vi "Test_waveform.vi"() -> ()   [LabVIEW 2017]
uses:
  Range_Shunt_selector.ctl
  <vilib>/Waveform/WDTFileIO.llb/ Write Waveform to File.vi
  <vilib>/Waveform/WDTFileIO.llb/Read Waveform from File.vi
  <vilib>/Utility/config.llb/Write Key (I32).vi
  <vilib>/Utility/config.llb/Write Key (Boolean).vi
  <vilib>/Utility/config.llb/Read Key (I32).vi
  <vilib>/Utility/config.llb/Read Key (Boolean).vi
  <vilib>/measure/madcrms.llb/Basic Averaged DC-RMS for 1 Chan.vi
  <resource>/objmgr/daqmx.rc
  <vilib>/Utility/config.llb/NI_LVConfig.lvlib
  <vilib>/measure/NI_MAPro.lvlib
panel:
  out "current time":timestamp
  out "Samples":i32=20000
  out "error out 3":errorcluster
  out "PhysicalChanName":tag
  out "DEV SN":u32 format="%.0x"
  out "mARange":dbl
  out "Boolean":bool
  out "DevSerialNum":u32
  in  "uA_bank0":dbl=1.5 format="%#_13g"
  out "Task out":refnum<k21>="Stop"
  out "Sample rate":dbl=20000.0 format="%#_13g"
  out "Clear":bool=TRUE
  out "Ver":string
  out "seconds since 1Jan1904":timestamp
  in  "Tab Control":enum32{"Current Tracking", "Logging"}(tab)
  out "Save":bool
  out "Total Time":string
  in  "Sampling Rate":T1(ring)
  out "out_range":bool
  in  "Save setting":bool
  out "PW_Source":bool
  out "EX_IN_INdicator":bool
  out "Lable.Unit_VOl_MA_UA":string
  in  "Ext PW Vol Monitor":bool
  out "POWER ON_OFF":bool
  out "vbat_lb":dbl format="%#_4f"
  in  "bypass Shunt":bool
  in  "Internal PW":bool
  in  "USB":tag="Dev1"
  out "schematic":bool
  in  "Save":bool
  in  "Load":bool
  in  "Calib":bool
  in  "Power ON/OFF":bool
  in  "Profile":enum16{"SAM", "DIANA", "Hi-POWER", "Other..."}(ring)
  in  "Take Picture":bool
  in  "Orginal":bool
  in  "Clear Graph":bool
  in  "ZOOM M1M2":bool
  in  "ZOOM -":bool
  in  "ZOOM +":bool
  in  "stop":bool
  out "Vbat":dbl format="%#.3f"
  in  "Measure":bool
  in  "Range - Shunts":T2
  out "PW_Internal_Source":dbl
  out "Min":dbl
  out "Max":dbl
  out "Delta(s)":sgl
  in  "Center":bool
  out "Avg":dbl
  out "Waveform_main":waveform(sgl)(graph)
  out "Waveform_sub":waveform(dbl)(graph)
  out "Average (uA)":dbl caption="Average (mA)" format="%#_6f"
  in  "Vout  - Vbat profile":enum16{"3.8VDC", "2.9VDC", "By Pass", "4.0VDC"}(ring)=enum."2.9VDC" caption="Vout  - Vbat"
  # "µPower kit for Wear OS Dev"
  # "Vbat"
  # "Vdut- Vbat"
  # "DUT"
  # "Rs"
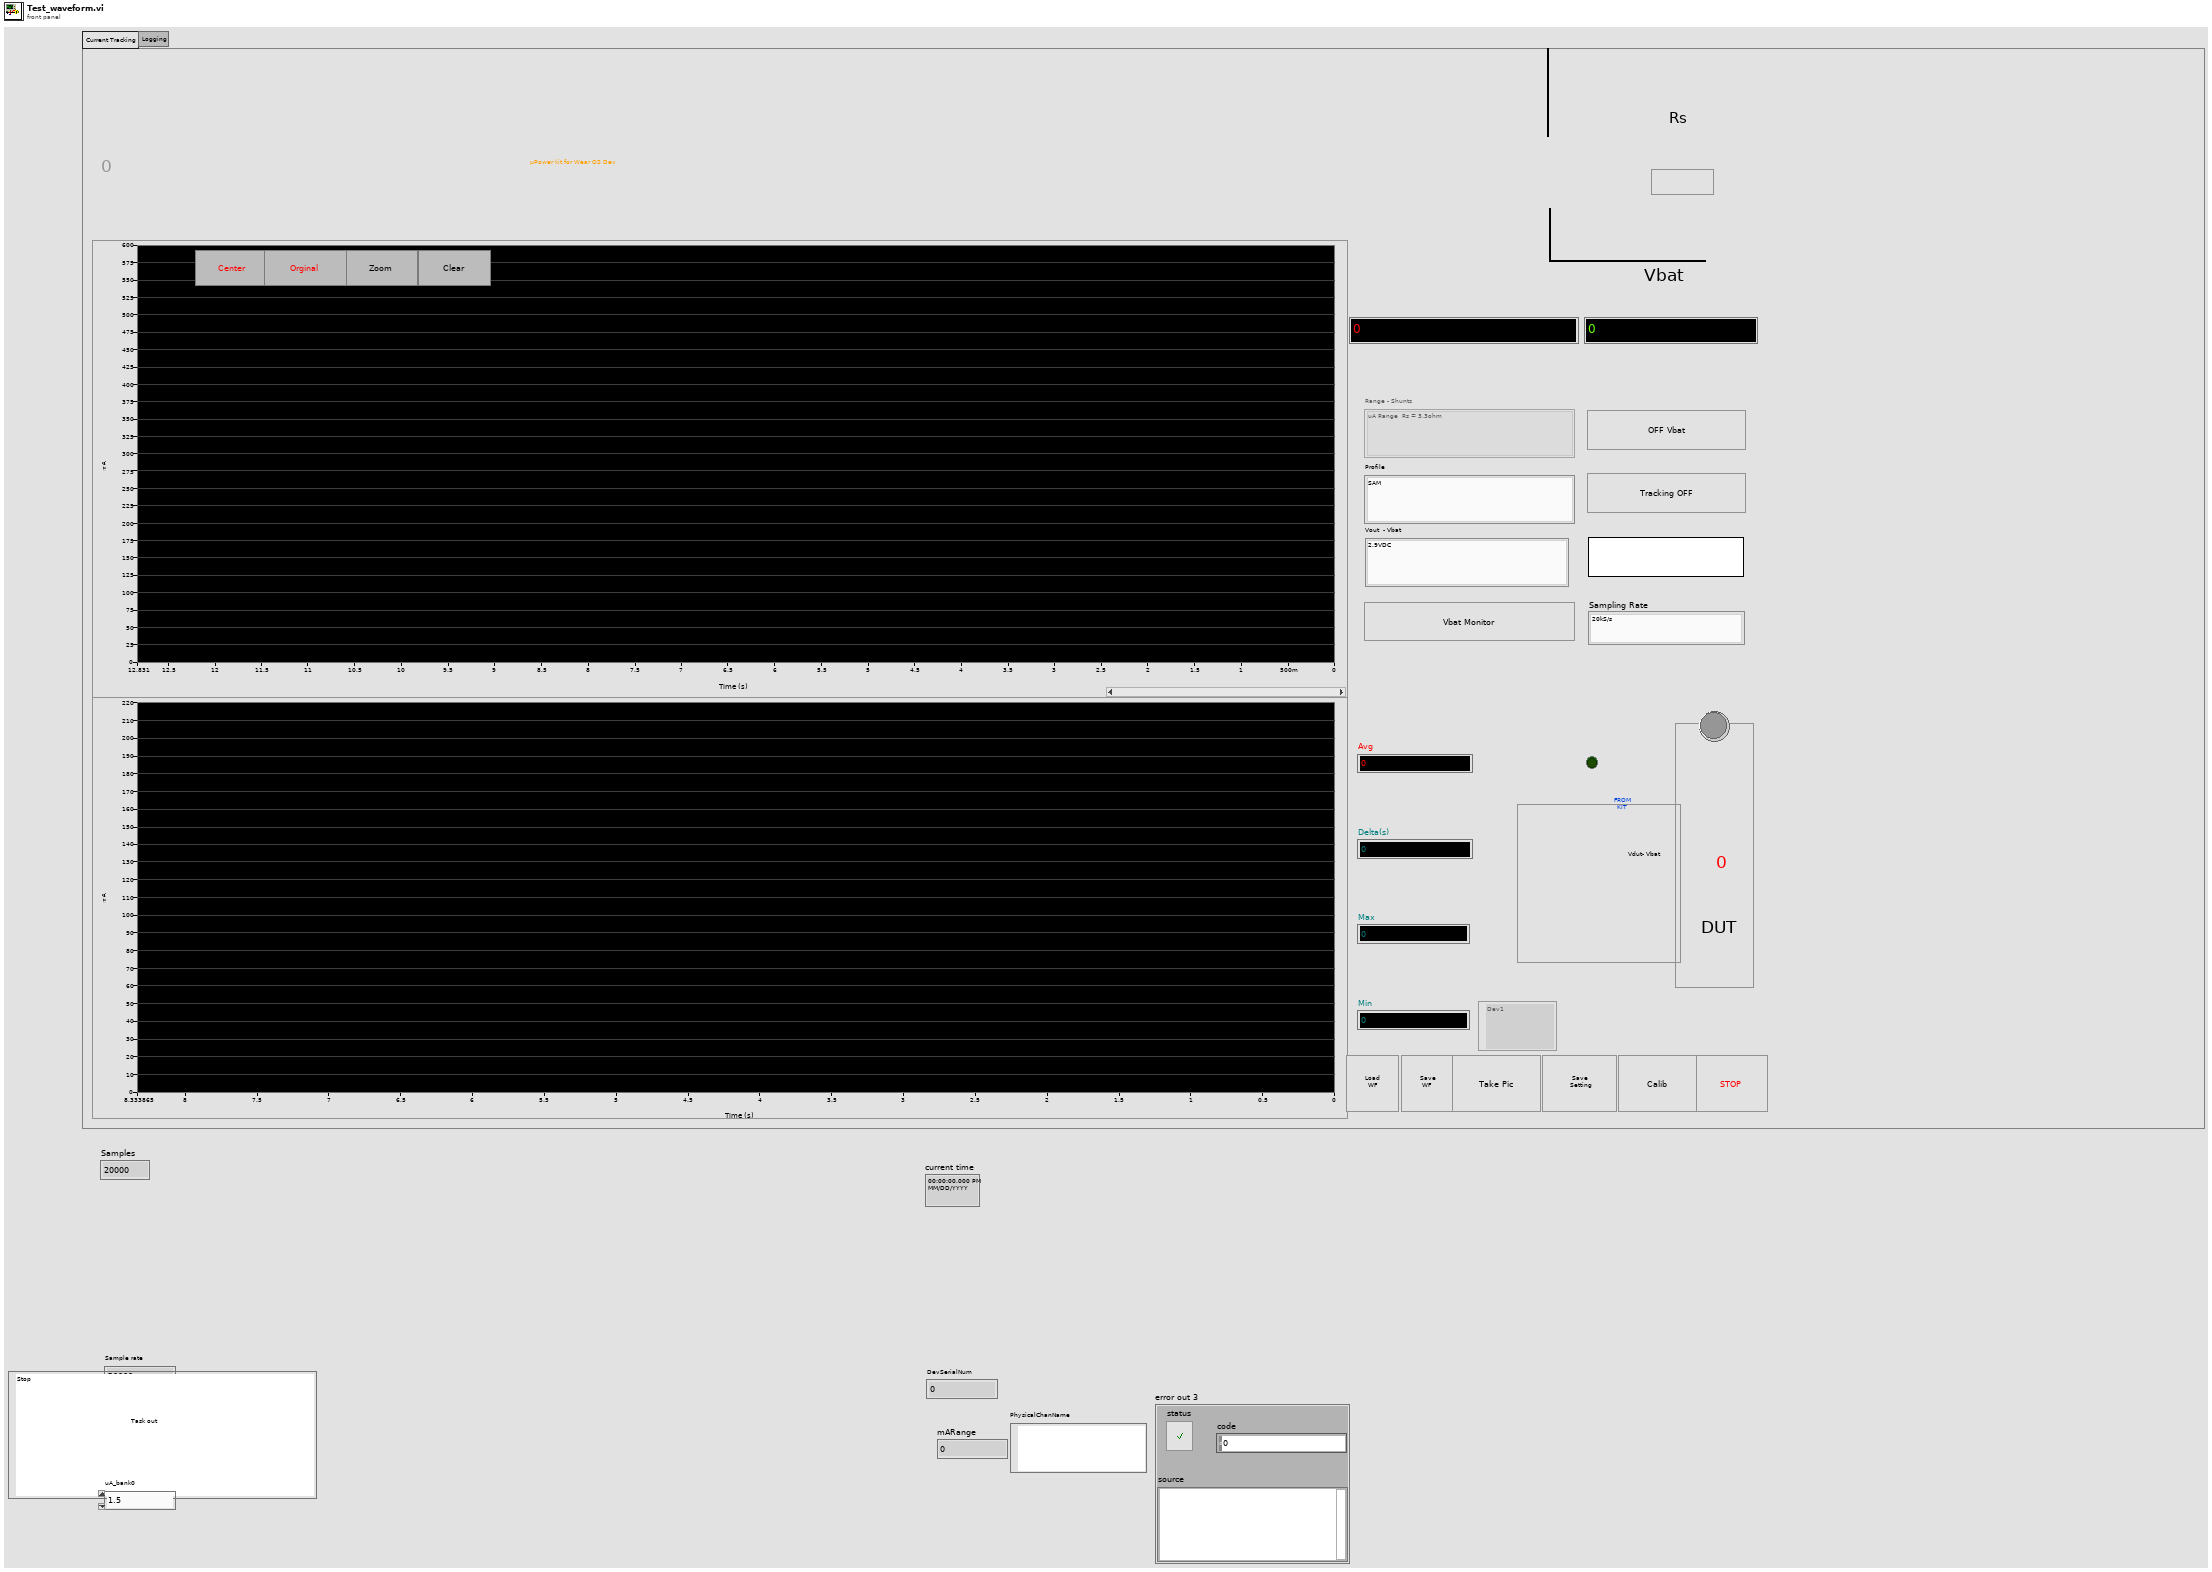
[diagram p1: front panel]
types:
  T1 = enum16{"20kS/s", "10kS/s", "5kS/s", "2kS/s", "1kS/s", "500S/s", "100S/s"}
  T2 = typedef "Range_Shunt_selector.ctl" = enum16{"uA Range  Rs = 3.3ohm", "mA Range Rs = 3.3ohm", "mA Range Rs = 1ohm", "mA Range Rs = 1ohm - X2"}
  T3 = enum8{"Enabled", "Disabled", "Disabled and Grayed Out"}
  T4 = typedef "NI_LVConfig.lvlib/Config Data RefNum.ctl" = refnum<k1>
  T5 = enum16{"Internal PW Source", "External PW Source"}
  T6 = enum16{"Turn On bypass - Off Shunt", "Turn Off bypass - On Shunt"}
  T7 = typedef "LVCursorListTypeDef.ctl" = cluster{"Name":string, "Color":u32, "Style":u8, "Point Style":u8, "Name Visible":bool, "Allow Drag":bool, "Cursor Mode":u32, "Plot":i32, "Index":i32, "Position":cluster{"X":dbl, "Y":dbl}, "X Scale":u32, "Y Scale":u32, "Watch Plots":i32[], "Watch All Plots":bool, "Plot Area":i32, "Label Offset":cluster{"X":dbl, "Y":dbl}}[]
  T8 = typedef "imagedata.ctl" = cluster{"image type":i32, "image depth":i32, "image":u8[], "mask":u8[], "colors":u32[], "Rectangle":cluster{"left":i16, "top":i16, "right":i16, "bottom":i16}}
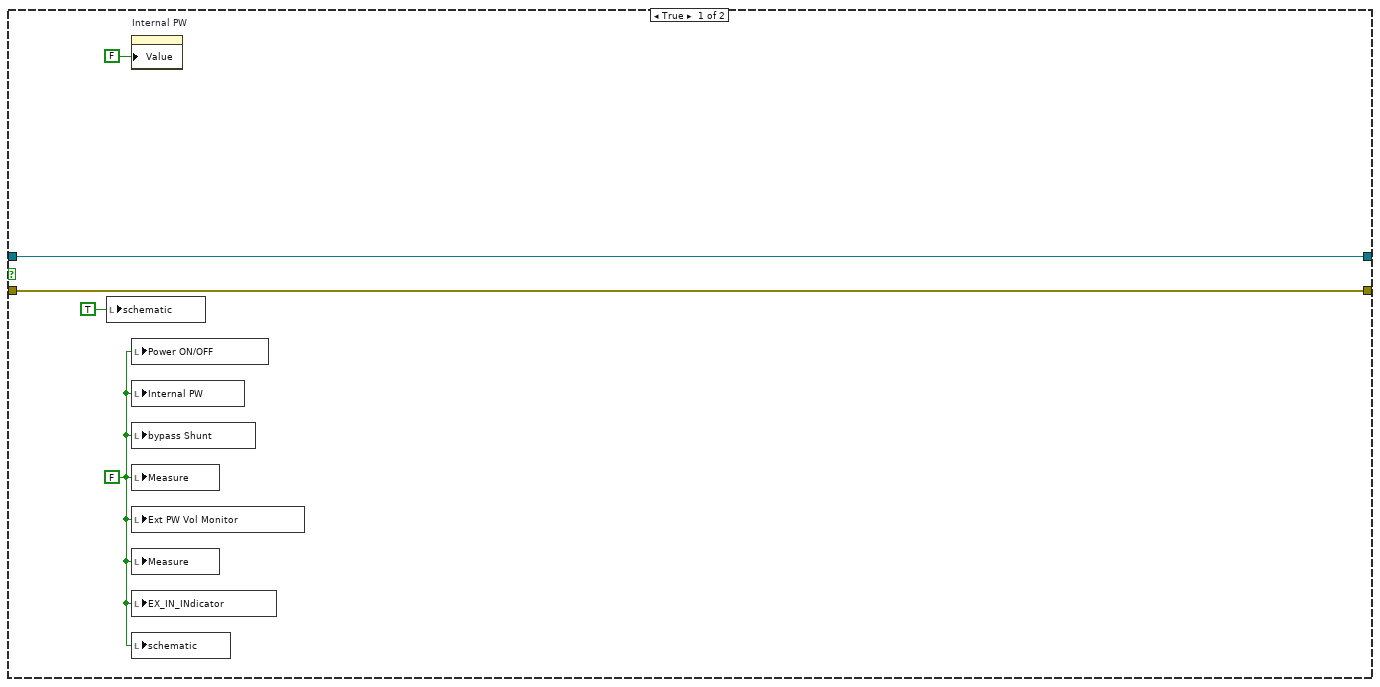
[diagram p2: hidden frame]
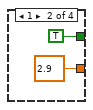
[diagram p3: hidden frame]
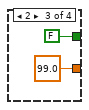
[diagram p4: hidden frame]
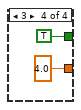
[diagram p5: hidden frame]
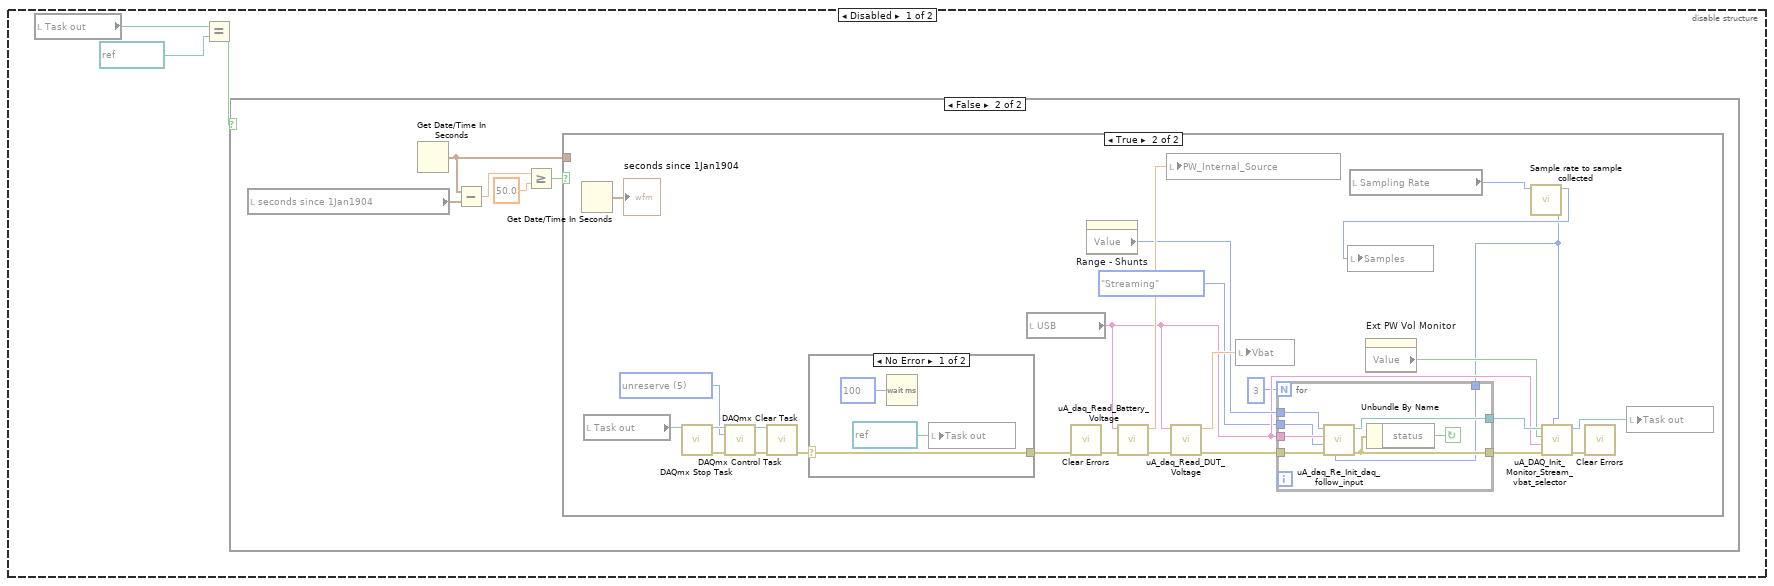
[diagram p7: hidden frame]
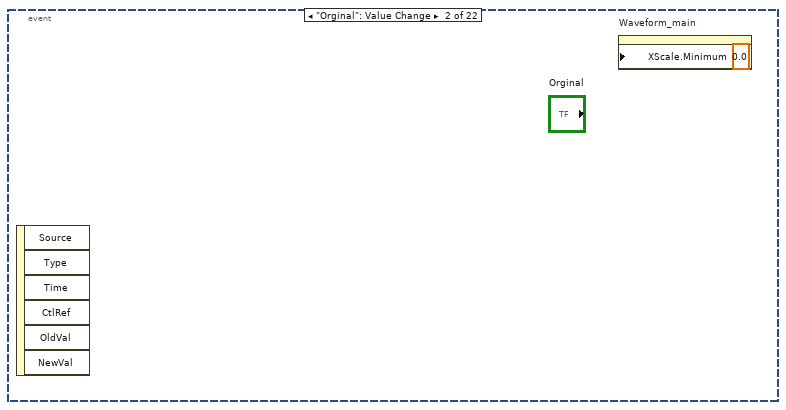
[diagram p12: hidden frame]
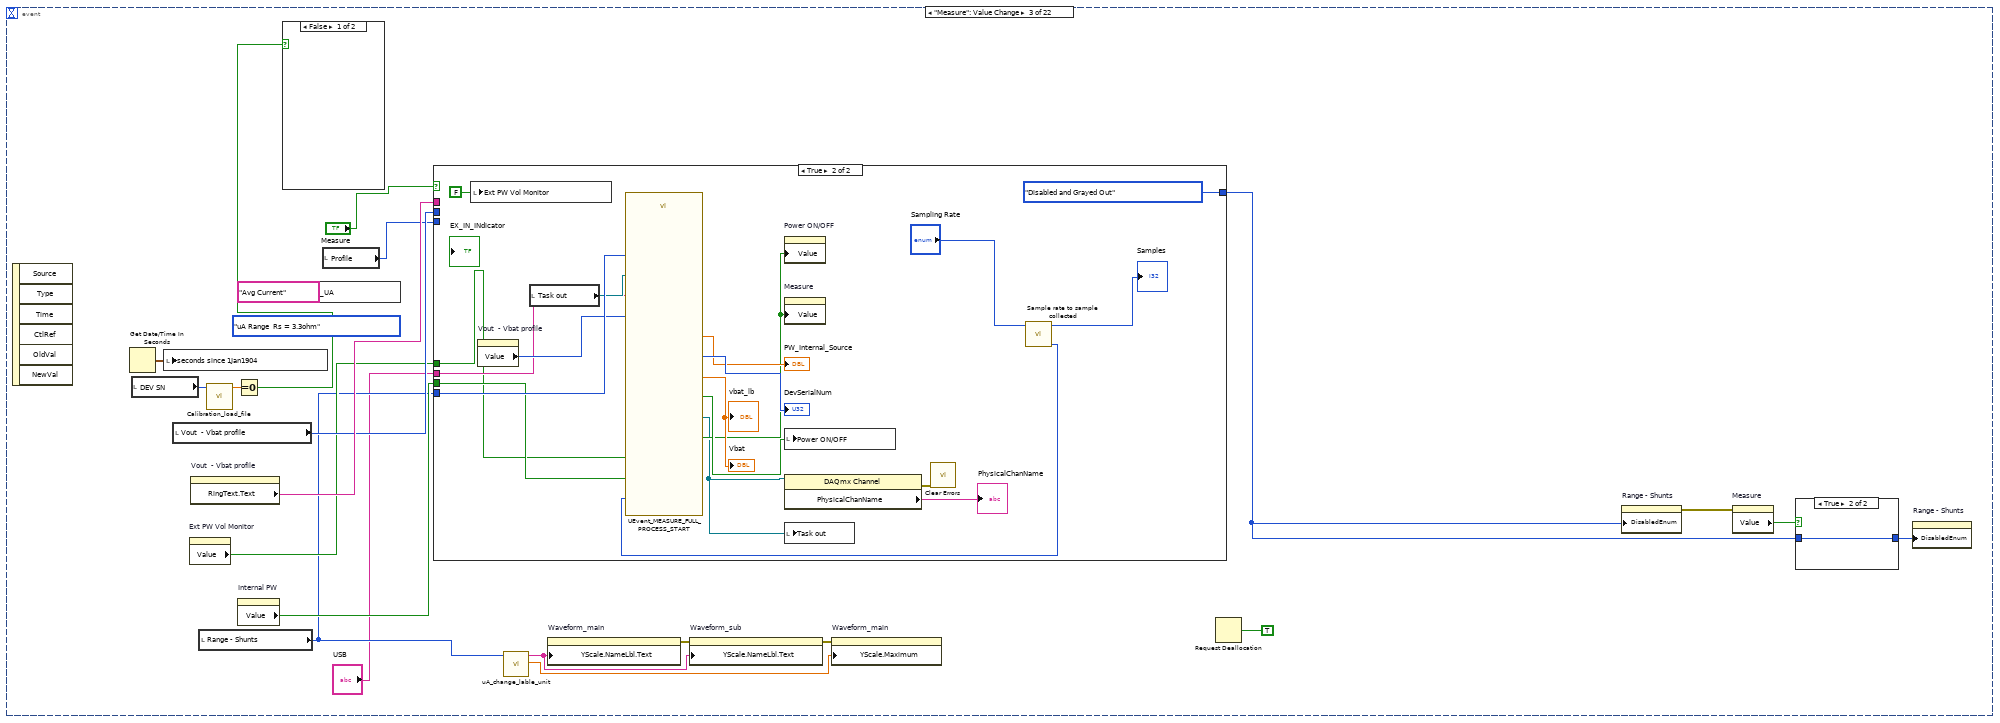
[diagram p13: hidden frame]
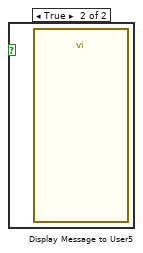
[diagram p14: hidden frame]
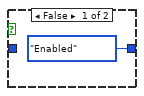
[diagram p15: hidden frame]
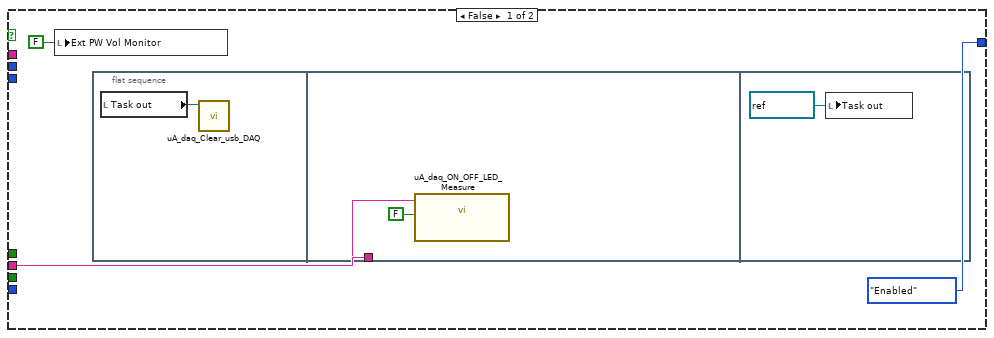
[diagram p16: hidden frame]
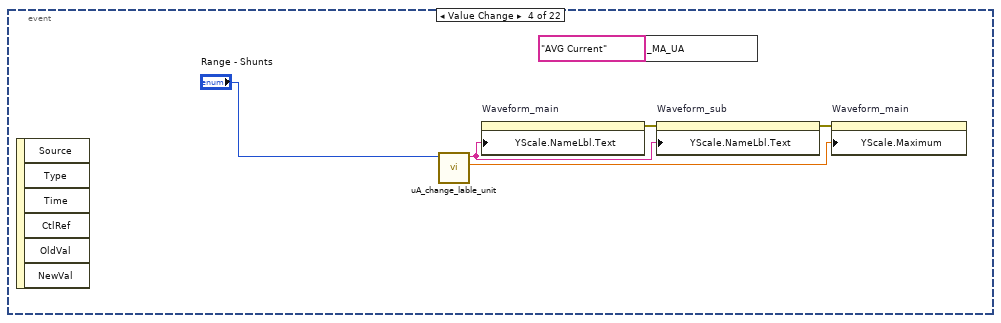
[diagram p17: hidden frame]
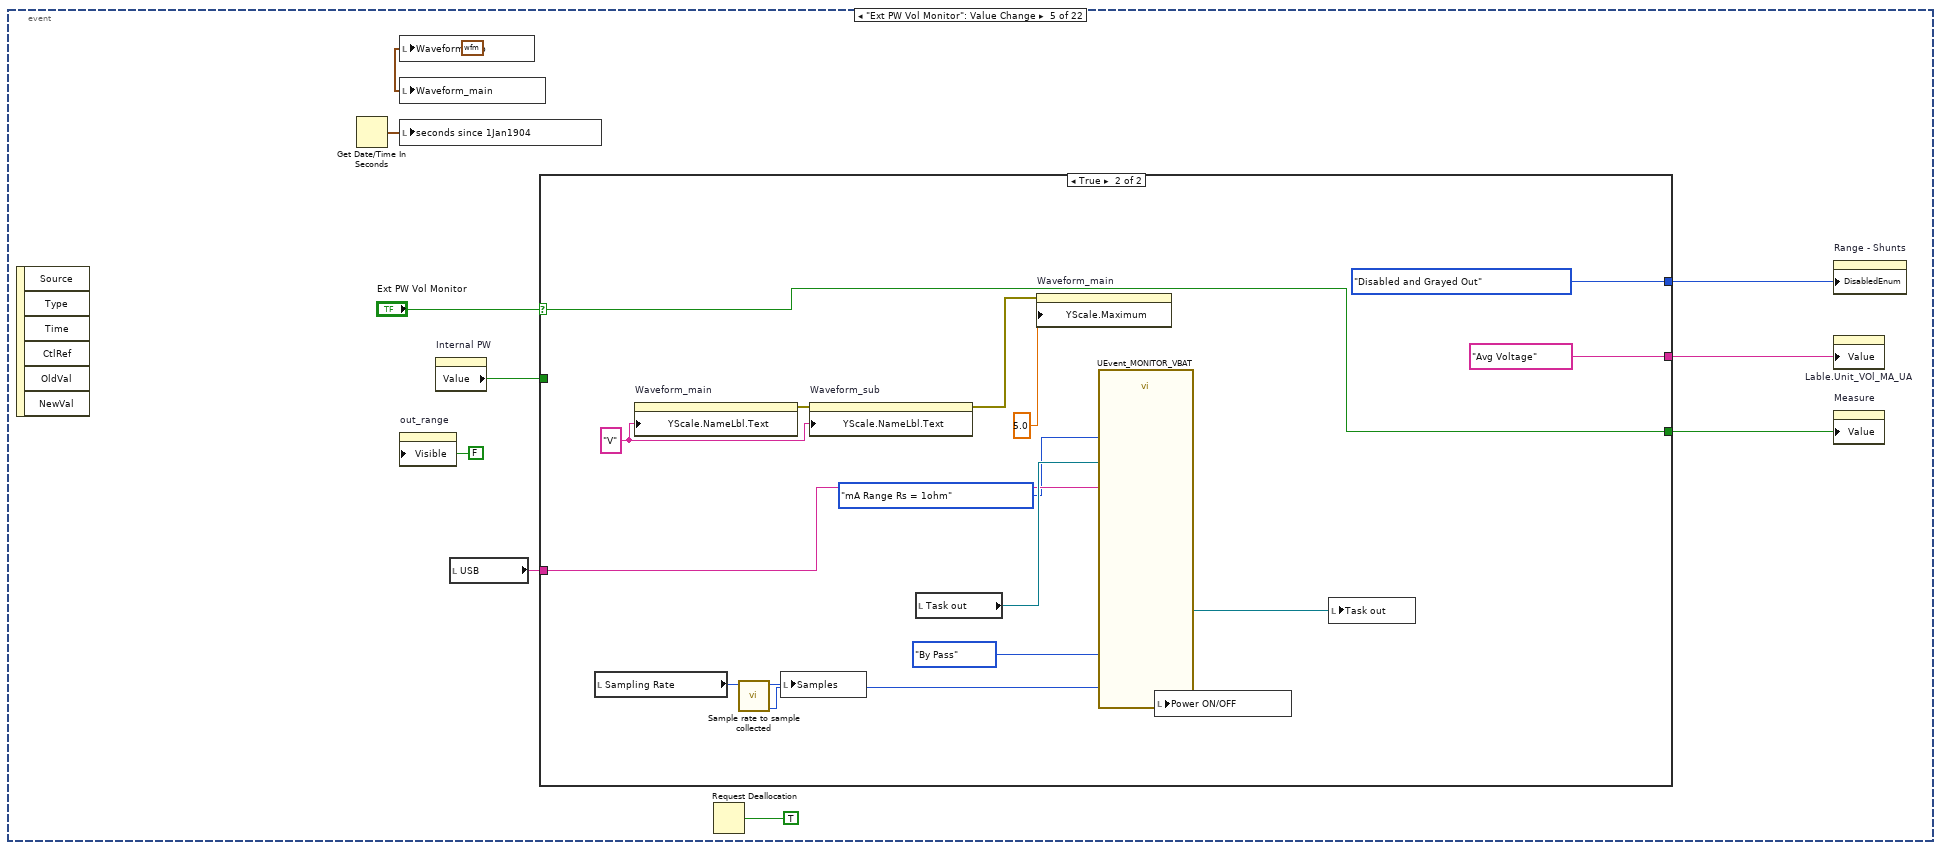
[diagram p18: hidden frame]
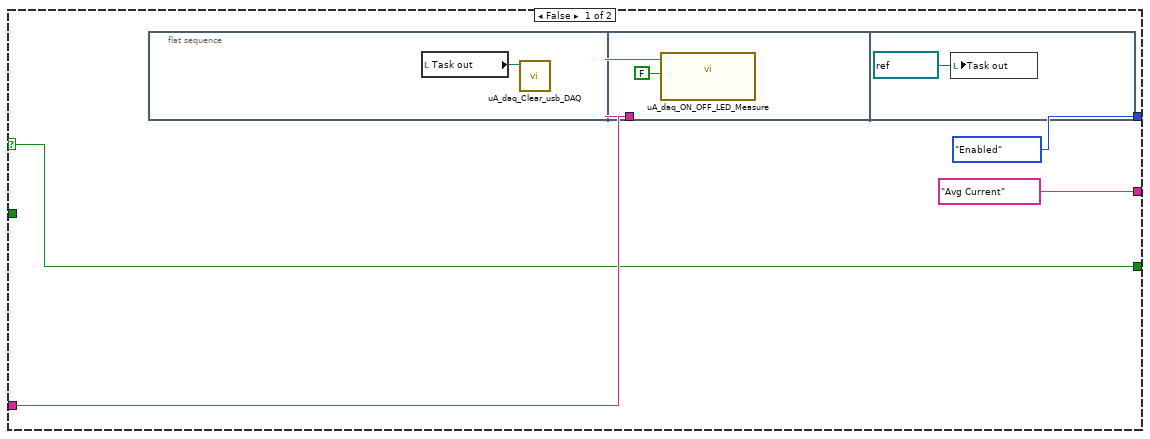
[diagram p19: hidden frame]
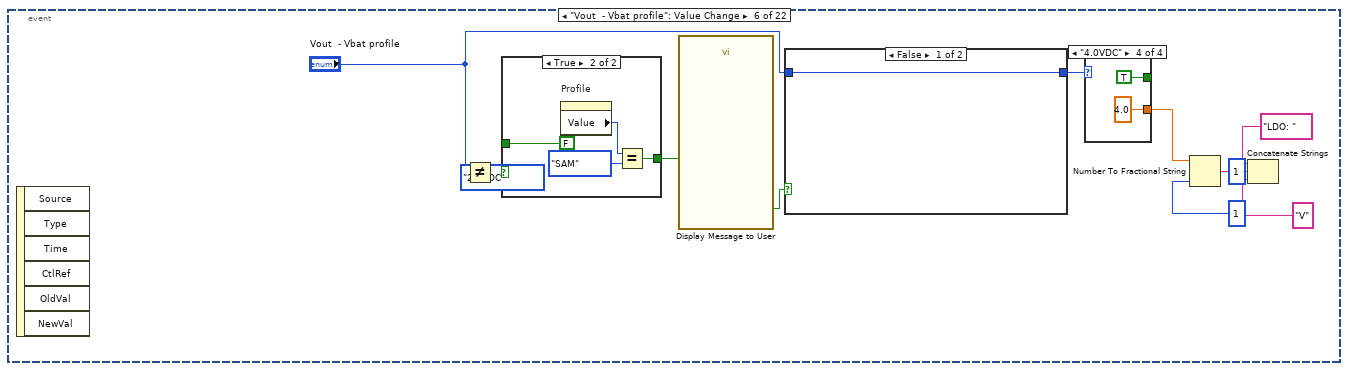
[diagram p20: hidden frame]
diagram:
  w2 = 24164516  # 1200s
  n1 = flat-sequence {
    tunnel: [w45] -> w5
    tunnel: [w48] -> w4
    frame #0 {
      w15 = TRUE ("s")
      w26 = FALSE ("Power ON/OFF")
      w45 = refnum<k21> "Stop" ("task out")
      n2 = property class="DAQmx System"() -> (error out=w39:errorcluster, "Device Names"=w40:tag[])  [unwired: 2 in, 1 out]
      n3 = property on="Range - Shunts" class="Enum (strict)"("DisabledEnum"=T3."Enabled" ("Disabled")) -> (error out=w8:errorcluster)  [unwired: 2 in, 1 out]
      n4 = local write "Vout  - Vbat profile"(enum16{"3.8VDC", "2.9VDC", "By Pass", "4.0VDC"}."By Pass" ("Vout  - Vbat profile")) -> ()
      n5 = local write "Profile"(enum16{"SAM", "DIANA", "Hi-POWER", "Other..."}."Hi-POWER" ("Profile")) -> ()
      n6 = for {
        tunnel: w40 -> [w97] mode=indexing
        shift-right: [w101] -> _
        shift-left: w39 -> [w102]
        tunnel: [w97] -> w38
        tunnel: [w96] -> w20
        stop <- w98 stop-if-true
        n7 = property class="DAQmx Device"(error in=w102, "Active Device"=w97) -> (error out=w101:errorcluster, "DevSerialNum"=w96:u32, "DevIsSimulated"=w100:bool)  [unwired: 1 in, 1 out]
        n8 = Equal?(x=w100, y=FALSE) -> (x = y?=w98:bool)
      }
      "DEV SN" <- w20
      n9 = local write "Power ON/OFF"(w26) -> ()
      n10 = local write "POWER ON_OFF"(w26) -> ()
      n11 = Select(t="Average (mA)" ("Caption.Text"), s=w15, f="Average (uA)" ("Caption.Text")) -> (s? t:f=w18:string)
      n12 = call <vilib>:"Application Directory.vi"() -> ("Application Directory"=w33:path)
      n13 = Select(t="mA" ("Caption.Text"), s=w15, f="uA" ("Caption.Text")) -> (s? t:f=w17:string)
      n14 = property on="out_range" class="Bool (strict)"(error in=w8, "Visible"=FALSE) -> (error out=w11:errorcluster)  [unwired: 1 in, 1 out]
      n15 = Build Path(base path=w33, name or relative path="Setting.cfg") -> (appended path=w31:path)
      n16 = property on="Average (uA)" class="DigNum (strict)"("Caption.Text"=w18) -> ()  [unwired: 2 in, 2 out]
      n17 = property on="Waveform_sub" class="WFGraph (strict)"("YScale.NameLbl.Text"=w17) -> ()  [unwired: 2 in, 2 out]
      n18 = property on="Waveform_main" class="WFGraph (strict)"("YScale.NameLbl.Text"=w17) -> ()  [unwired: 2 in, 2 out]
      n19 = call <vilib>:"Open Config Data.vi"("configuration file path"=w31) -> ("error out"=w27:errorcluster, "file created?"=w34:bool, "refnum"=w30:T4)  [unwired: 8 in]
      n20 = property on="Ext PW Vol Monitor" class="Bool (strict)"(error in=w11, "Value"=FALSE ("Record uA & Vbat")) -> (error out=w10:errorcluster)  [unwired: 1 in, 1 out]
      n21 = case shown="False" w34 {
        tunnel: w27 -> [w57 w87]
        tunnel: [w57 w82] -> w28
        tunnel: [w56 w81] -> w29
        tunnel: w30 -> [w56 w70]
        frame True {
          w55 = FALSE ("Measure")
          n22 = local write "schematic"(TRUE ("schematic")) -> ()
          n23 = property on="Internal PW" class="Bool (strict)"("Value"=FALSE ("Internal PW")) -> ()  [unwired: 2 in, 2 out]
          n24 = local write "Power ON/OFF"(w55) -> ()
          n25 = local write "Internal PW"(w55) -> ()
          n26 = local write "bypass Shunt"(w55) -> ()
          n27 = local write "Measure"(w55) -> ()
          n28 = local write "Ext PW Vol Monitor"(w55) -> ()
          n29 = local write "Measure"(w55) -> ()
          n30 = local write "EX_IN_INdicator"(w55) -> ()
          n31 = local write "schematic"(w55) -> ()
        }
        frame False {
          (unwired) FALSE ("Visible")
          w58 = TRUE
          w71 = "SETTING" ("section")
          n32 = Not(x=w58) -> ()  [unwired: 1 out]
          n33 = local write "Internal PW"(w58) -> ()
          n34 = local write "EX_IN_INdicator"(w58) -> ()
          n35 = local write "Vout  - Vbat profile"(enum16{"3.8VDC", "2.9VDC", "By Pass", "4.0VDC"}."By Pass" ("Vout  - Vbat profile")) -> ()
          n36 = local write "Profile"(enum16{"SAM", "DIANA", "Hi-POWER", "Other..."}."Hi-POWER" ("Profile")) -> ()
          n37 = call-poly <vilib>:"Read Key.vi"("section"=w71, "error in (no error)"=w87, "key"="Range - Shunts", "refnum"=w70) -> ("error out"=w86:errorcluster, "refnum out"=w73:T4)  [unwired: 4 in, 2 out]
          n38 = local write "Range - Shunts"(Range_Shunt_selector."mA Range Rs = 1ohm" ("Range - Shunts")) -> ()
          n39 = call-poly <vilib>:"Read Key.vi"("section"=w71, "error in (no error)"=w86, "key"="Profile", "refnum"=w73) -> ("error out"=w85:errorcluster, "refnum out"=w72:T4)  [unwired: 4 in, 2 out]
          n40 = call-poly <vilib>:"Read Key.vi"("section"=w71, "error in (no error)"=w85, "key"="Vout  - Vbat profile", "refnum"=w72) -> ("error out"=w84:errorcluster, "value"=w62:i32, "refnum out"=w74:T4)  [unwired: 4 in, 1 out]
          n41 = case shown="0, Default" w62 {
            tunnel: [3.8 2.9 99.0 4.0] -> w66
            tunnel: [TRUE ("Visible") TRUE ("Visible") FALSE ("Visible") TRUE ("Visible")] -> _
            frame 0, Default {
            }
            frame 1 {
            }
            frame 2 {
            }
            frame 3 {
            }
          }
          n42 = call-poly <vilib>:"Read Key.vi"("section"=w71, "error in (no error)"=w84, "key"="Internal PW", "refnum"=w74) -> ("error out"=w83:errorcluster, "refnum out"=w75:T4)  [unwired: 4 in, 2 out]
          n43 = call-poly <vilib>:"Read Key.vi"("section"=w71, "error in (no error)"=w83, "key"="bypass Shunt", "refnum"=w75) -> ("error out"=w82:errorcluster, "value"=w69:bool, "refnum out"=w81:T4)  [unwired: 4 in, 1 out]
          n44 = local write "bypass Shunt"(w69) -> ()
          n45 = Number To Fractional String(number=w66, width (-)=i16 1, precision (6)=i16 1) -> (F-format string=w63:string)  [unwired: 1 in]
          n46 = Concatenate Strings("LDO: " ("string"), w63, "V" ("string")) -> ()  [unwired: 1 out]
        }
      }
      n47 = local write "USB"(w38) -> ()
      n48 = property on="out_range" class="Bool (strict)"(error in=w10, "Visible"=FALSE) -> (error out=w9:errorcluster)  [unwired: 1 in, 1 out]
      n49 = call "Calibration_load_file.vi"("DEV SN"=w20) -> ("Calib value-mA"=→"mARange":dbl, "Calib value-uA"=w21:dbl)  [unwired: 8 in]
      n50 = local write "uA_bank0"(w21) -> ()
      n51 = call <vilib>:"Application Directory.vi"() -> ("Application Directory"=w47:path)
      n52 = call "uA_build_version.vi"("error in (no error)"=w9, "name or relative path"="uPower_kit_wear_os.exe", "path"=w47) -> ("error out"=w44:errorcluster, "FileVersion"=w43:string)  [unwired: 6 in, 1 out]
      n53 = case shown="Error" w44 {
        selector: w44 -> [_ w105]
        tunnel: w43 -> [w103 _]
        tunnel: [w103 "" ("FileVersion")] -> w42
        frame No Error {
        }
        frame Error {
          n54 = call <vilib>:"Clear Errors.vi"("error in (no error)"=w105) -> ()  [unwired: 5 in, 2 out]
        }
      }
      "Ver" <- w42
      n55 = local write "Measure"(FALSE ("Measure")) -> ()
      n56 = local write "schematic"(TRUE ("schematic")) -> ()
      n57 = call <vilib>:"Close Config Data.vi"("error in (no error)"=w28, "refnum"=w29) -> ()  [unwired: 8 in, 2 out]
      n58 = Obtain Queue(name (unnamed)="Data", element data type=waveform(sgl) {"t0"=timestamp(0 s since 1904-01-01), "dt"=1.0, "Y"=[]} ("Waveform Chart 2")) -> (queue out=w48:refnum<queue>)  [unwired: 3 in, 2 out]
      "Clear" <- FALSE ("Clear")
      "Sample rate" <- 20000.0 ("Sample rate")
      "Task out" <- w45
    }
  }
  n59 = Multiply(x=w2, y=4) -> (x*y=w1:i32)
  n60 = while {
    stop <- FALSE stop-if-true
    n61 = event shown="[0] Timeout" {
      selector: _ -> [_ _ _ _ _ _ _ _ _ _ _ _ _ _ _ _ _ _ _ _ _ _]
      dyn-events: _ -> [_ _ _ _ _ _ _ _ _ _ _ _ _ _ _ _ _ _ _ _ _ _]
      timeout: 400 -> [_ _ _ _ _ _ _ _ _ _ _ _ _ _ _ _ _ _ _ _ _ _]
      event Timeout {
        n62 = event-data() -> ()  [unwired: 1 in, 3 out]
        n63 = disable-structure shown="Enabled" {
          frame Disabled {
            n64 = local read "Task out"() -> (w109:refnum<k21>)
            n65 = Equal?(x=w109, y=refnum<k21> "Stop") -> (x = y?=w110:bool)
            n66 = case shown="False" w110 {
              frame True {
              }
              frame False {
                n67 = local read "seconds since 1Jan1904"() -> (w112:timestamp)
                n68 = Get Date/Time In Seconds() -> (seconds since 1Jan1904=w113:timestamp)
                n69 = Subtract(x=w113, y=w112) -> (x-y=w116:dbl)
                n70 = Greater Or Equal?(x=w116, y=50.0) -> (x >= y?=w114:bool)
                n71 = case shown="True" w114 {
                  tunnel: w113 -> [_ _]
                  frame False {
                  }
                  frame True {
                    w126 = 5 items=["verify"=2, "reserve"=4, "commit"=3, "unreserve"=5, "abort"=6] ("action")
                    n72 = Get Date/Time In Seconds() -> (seconds since 1Jan1904=→"seconds since 1Jan1904":timestamp)
                    n73 = local read "Task out"() -> (w141:refnum<k21>)
                    n74 = call <vilib>:"DAQmx Stop Task.vi"("task/channels in"=w141) -> ("task out"=w130:refnum<k21>, "error out"=w128:errorcluster)  [unwired: 13 in]
                    n75 = call <vilib>:"DAQmx Control Task.vi"("task/channels in"=w130, "action"=w126, "error in"=w128) -> ("task out"=w129:refnum<k21>, "error out"=w127:errorcluster)  [unwired: 11 in]
                    n76 = call <vilib>:"DAQmx Clear Task.vi"("task in"=w129, "error in"=w127) -> ("error out"=w122:errorcluster)  [unwired: 13 in]
                    n77 = case shown="No Error" w122 {
                      selector: w122 -> [w144 w146]
                      tunnel: [w144 w146] -> w121
                      frame No Error {
                        n78 = Wait (ms)(milliseconds to wait=u32 100) -> ()  [unwired: 1 out]
                        n79 = local write "Task out"(refnum<k21> "Stop" ("Task out")) -> ()
                      }
                      frame Error {
                      }
                    }
                    n80 = local read "USB"() -> (w132:tag)
                    n81 = call <vilib>:"Clear Errors.vi"("error in (no error)"=w121) -> ("error out"=w140:errorcluster)  [unwired: 5 in, 1 out]
                    n82 = property on="Range - Shunts" class="Enum (strict)"() -> ("Value"=w136:T2)  [unwired: 2 in, 2 out]
                    n83 = call "uA_daq_Read_Battery_Voltage.vi"("error in"=w140, "USB DAQ"=w132) -> ("error out"=w137:errorcluster, "Battery_Voltage"=w139:dbl)  [unwired: 8 in]
                    n84 = local write "PW_Internal_Source"(w139) -> ()
                    n85 = call "uA_daq_Read_DUT_Voltage.vi"("error in"=w137, "USB DAQ"=w132) -> ("error out"=w125:errorcluster, "DUT_Voltage"=w138:dbl)  [unwired: 8 in]
                    n86 = local write "Vbat"(w138) -> ()
                    n87 = local read "Sampling Rate"() -> (w118:T1)
                    n88 = property on="Ext PW Vol Monitor" class="Bool (strict)"() -> ("Value"=w133:bool)  [unwired: 2 in, 2 out]
                    n89 = call "Sample rate to sample collected.vi"("Sampling Rate _menu"=w118) -> ("Sample_rate"=w117:u32, "Sample"=w119:i32)  [unwired: 9 in]
                    n90 = for {
                      N: 3 -> [_]
                      tunnel: w136 -> [w154]
                      tunnel: [w153] -> w135
                      tunnel: w132 -> [w152]
                      tunnel: enum16{"Streaming", "Read All", "Stop"}."Streaming" ("Acquire Mode") -> [w150]
                      tunnel: w125 -> [w151]
                      tunnel: [w149] -> w131
                      tunnel: w117 -> [w147]
                      stop <- w148 continue-if-true
                      n91 = call "uA_daq_Re_Init_daq_follow_input.vi"("rate"=w147, "error in (no error)"=w151, "Acquire Mode"=w150, "USB"=w152, "Range_shunt"=w154) -> ("error out"=w149:errorcluster, "Refnum out"=w153:refnum<k21>)  [unwired: 5 in]
                      n92 = Unbundle By Name(w149) -> ("status"=w148:bool)
                    }
                    n93 = local write "Samples"(w119) -> ()
                    n94 = call "uA_DAQ_Init_Monitor_Stream_vbat_selector.vi"("Sample rate"=w117, "error in (no error)"=w131, "USB"=w132, "Ext PW Vol Monitor"=w133, "Refnum in"=w135) -> ("error out"=w120:errorcluster, "Refnum out"=w134:refnum<k21>)  [unwired: 5 in]
                    n95 = call <vilib>:"Clear Errors.vi"("error in (no error)"=w120) -> ()  [unwired: 5 in, 2 out]
                    n96 = local write "Task out"(w134) -> ()
                  }
                }
              }
            }
          }
          frame Enabled {
            n97 = local read "current time"() -> (w156:timestamp)
            n98 = Get Date/Time In Seconds() -> (seconds since 1Jan1904=w157:timestamp)
            n99 = Subtract(x=w157, y=w156) -> (x-y=w160:dbl)
            n100 = Greater?(x=w160, y=60.0) -> (0:w158:bool)
            n101 = case shown="True" w158 {
              tunnel: w157 -> [_ w165]
              frame False {
              }
              frame True {
                n102 = call <vilib>:"Application Directory.vi"() -> ("Application Directory"=w168:path)
                n103 = Build Path(base path=w168, name or relative path="datalog.dlog" ("pattern label")) -> (appended path=w163:path)
                n104 = Delete(path (use dialog)=w163) -> (error out=w162:errorcluster)  [unwired: 4 in, 2 out]
                n105 = local write "Save"(TRUE ("Save")) -> ()
                n106 = local read "Waveform_main"() -> (w164:waveform(sgl))
                n107 = call-poly <vilib>:"Write Waveforms to File.vi"("error in (no error)"=w162, "append to file? (new file:F)"=FALSE, "waveform"=w164, "file path (dialog if empty)"=w163) -> ()  [unwired: 6 in, 2 out]
                "current time" <- w165
              }
            }
            "Save" <- FALSE ("Save")
          }
        }
        n108 = local read "Vbat"() -> (w108:dbl)
        n109 = local write "vbat_lb"(w108) -> ()
      }
      event "Orginal": Value Change {
        n110 = event-data() -> ()  [unwired: 1 in, 6 out]
        n111 = property on="Waveform_main" class="WFGraph (strict)"("XScale.Minimum"=0.0 ("X Scale.Range:Minimum")) -> ()  [unwired: 2 in, 2 out]
      }
      event "Measure": Value Change {
        (unwired) Range_Shunt_selector."uA Range  Rs = 3.3ohm" ("Range - Shunts")
        n112 = event-data() -> ()  [unwired: 1 in, 6 out]
        n113 = Get Date/Time In Seconds() -> (seconds since 1Jan1904=w190:timestamp)
        n114 = local read "DEV SN"() -> (w172:u32)
        n115 = local write "seconds since 1Jan1904"(w190) -> ()
        n116 = local read "Vout  - Vbat profile"() -> (w187:enum16{"3.8VDC", "2.9VDC", "By Pass", "4.0VDC"})
        n117 = property on="Ext PW Vol Monitor" class="Bool (strict)"() -> ("Value"=w180:bool)  [unwired: 2 in, 2 out]
        n118 = property on="Vout  - Vbat profile" class="Enum (strict)"() -> ("RingText.Text"=w188:string)  [unwired: 2 in, 2 out]
        n119 = local read "Range - Shunts"() -> (w178:T2)
        n120 = call "Calibration_load_file.vi"("DEV SN"=w172) -> ("Calib value-uA"=w171:dbl)  [unwired: 8 in, 1 out]
        n121 = Equal To 0?(x=w171) -> (x = 0?=w170:bool)
        n122 = property on="Internal PW" class="Bool (strict)"() -> ("Value"=w181:bool)  [unwired: 2 in, 2 out]
        n123 = local write "Lable.Unit_VOl_MA_UA"("Avg Current" ("Lable.Unit_VOl_MA_UA")) -> ()
        n124 = case shown="False" w170 {
          frame False {
          }
          frame True {
            n125 = call "Display Message to User5"() -> ()  [unwired: 10 in, 2 out]
          }
        }
        n126 = local read "Profile"() -> (w186:enum16{"SAM", "DIANA", "Hi-POWER", "Other..."})
        n127 = case shown="True" "Measure" {
          tunnel: w188 -> [_ _]
          tunnel: w187 -> [_ _]
          tunnel: w186 -> [_ _]
          tunnel: w178 -> [_ w216]
          tunnel: w181 -> [_ w212]
          tunnel: "USB" -> [w195 w210]
          tunnel: w180 -> [_ w207]
          tunnel: [T3."Enabled" ("Disabled") T3."Disabled and Grayed Out" ("Disabled")] -> w174
          frame False {
            n128 = local write "Ext PW Vol Monitor"(FALSE ("Ext PW Vol Monitor")) -> ()
            n129 = flat-sequence {
              tunnel: w195 -> [w199]
              frame #0 {
                n130 = local read "Task out"() -> (w197:refnum<k21>)
                n131 = call "uA_daq_Clear_usb_DAQ.vi"("Refnum in"=w197) -> ()  [unwired: 11 in]
              }
              frame #1 {
                n132 = call "uA_daq_ON_OFF_LED_Measure.vi"("LED_meas"=FALSE ("Boolean"), "USB"=w199) -> ()  [unwired: 9 in, 1 out]
              }
              frame #2 {
                n133 = local write "Task out"(refnum<k21> "Stop" ("Refnum out")) -> ()
              }
            }
          }
          frame True {
            n134 = local write "Ext PW Vol Monitor"(FALSE ("Ext PW Vol Monitor")) -> ()
            n135 = property on="Vout  - Vbat profile" class="Enum (strict)"() -> ("Value"=w213:enum16{"3.8VDC", "2.9VDC", "By Pass", "4.0VDC"})  [unwired: 2 in, 2 out]
            n136 = local read "Task out"() -> (w215:refnum<k21>)
            n137 = call "Sample rate to sample collected.vi"("Sampling Rate _menu"="Sampling Rate") -> ("Sample_rate"=w201:u32, "Sample"=→"Samples":i32)  [unwired: 9 in]
            n138 = call "UEvent_MEASURE_FULL_PROCESS_START.vi"("Refnum in"=w215, "Range - Shunts"=w216, "Ext PW Vol Monitor"=w207, "USB"=w210, "Internal/external Power"=w212, "Vout  - Vbat profile"=w213, "Sample rate"=w201) -> ("DevSerialNum"=→"DevSerialNum":u32, "Power ON/OFF"=w218:bool, "Refnum out"=w209:refnum<k21>, "Battery_Voltage"=→"PW_Internal_Source":dbl, "DUT_Voltage"=→"Vbat" →"vbat_lb":dbl, "Measure indicator"=w211:bool)  [unwired: 2 in, 1 out]
            n139 = property on="Power ON/OFF" class="Bool (strict)"("Value"=w211) -> ()  [unwired: 2 in, 2 out]
            n140 = property on="Measure" class="Bool (strict)"("Value"=w211) -> ()  [unwired: 2 in, 2 out]
            n141 = local write "Power ON/OFF"(w218) -> ()
            n142 = property class="DAQmx Channel"(reference=w209) -> (error out=w206:errorcluster, "PhysicalChanName"=→"PhysicalChanName":tag)  [unwired: 1 in, 1 out]
            n143 = local write "Task out"(w209) -> ()
            n144 = call <vilib>:"Clear Errors.vi"("error in (no error)"=w206) -> ()  [unwired: 5 in, 2 out]
          }
        }
        n145 = call "uA_change_lable_unit.vi"("Range - Shunts"=w178) -> ("Y_scale"=w183:dbl, "unit"=w182:string)  [unwired: 8 in, 1 out]
        n146 = property on="Waveform_main" class="WFGraph (strict)"("YScale.NameLbl.Text"=w182) -> (error out=w185:errorcluster)  [unwired: 2 in, 1 out]
        n147 = property on="Waveform_sub" class="WFGraph (strict)"(error in=w185, "YScale.NameLbl.Text"=w182) -> (error out=w184:errorcluster)  [unwired: 1 in, 1 out]
        n148 = property on="Waveform_main" class="WFGraph (strict)"(error in=w184, "YScale.Maximum"=w183) -> ()  [unwired: 1 in, 2 out]
        n149 = Request Deallocation(TRUE ("flag")) -> ()
        n150 = property on="Range - Shunts" class="Enum (strict)"("DisabledEnum"=w174) -> (error out=w177:errorcluster)  [unwired: 2 in, 1 out]
        n151 = property on="Measure" class="Bool (strict)"(error in=w177) -> ("Value"=w176:bool)  [unwired: 1 in, 2 out]
        n152 = case shown="True" w176 {
          tunnel: [T3."Enabled" ("Disabled") w193] -> w175
          tunnel: w174 -> [_ w193]
          frame False {
          }
          frame True {
          }
        }
        n153 = property on="Range - Shunts" class="Enum (strict)"("DisabledEnum"=w175) -> ()  [unwired: 2 in, 2 out]
      }
      event Value Change {
        n154 = event-data() -> ()  [unwired: 1 in, 6 out]
        n155 = call "uA_change_lable_unit.vi"("Range - Shunts"="Range - Shunts") -> ("Y_scale"=w223:dbl, "unit"=w222:string)  [unwired: 8 in, 1 out]
        n156 = property on="Waveform_main" class="WFGraph (strict)"("YScale.NameLbl.Text"=w222) -> (error out=w225:errorcluster)  [unwired: 2 in, 1 out]
        n157 = local write "Lable.Unit_VOl_MA_UA"("AVG Current" ("Lable.Unit_VOl_MA_UA")) -> ()
        n158 = property on="Waveform_sub" class="WFGraph (strict)"(error in=w225, "YScale.NameLbl.Text"=w222) -> (error out=w224:errorcluster)  [unwired: 1 in, 1 out]
        n159 = property on="Waveform_main" class="WFGraph (strict)"(error in=w224, "YScale.Maximum"=w223) -> ()  [unwired: 1 in, 2 out]
      }
      event "Ext PW Vol Monitor": Value Change {
        w228 = waveform(sgl) {"t0"=timestamp(0 s since 1904-01-01), "dt"=1.0, "Y"=[]} ("Waveform_main")
        n160 = event-data() -> ()  [unwired: 1 in, 6 out]
        n161 = Get Date/Time In Seconds() -> (seconds since 1Jan1904=w234:timestamp)
        n162 = local write "Waveform_sub"(w228) -> ()
        n163 = local write "Waveform_main"(w228) -> ()
        n164 = local write "seconds since 1Jan1904"(w234) -> ()
        n165 = property on="out_range" class="Bool (strict)"("Visible"=FALSE) -> ()  [unwired: 2 in, 2 out]
        n166 = property on="Internal PW" class="Bool (strict)"() -> ("Value"=w233:bool)  [unwired: 2 in, 2 out]
        n167 = local read "USB"() -> (w231:tag)
        n168 = case shown="True" "Ext PW Vol Monitor" {
          selector: "Ext PW Vol Monitor" -> [w238 w256]
          tunnel: w233 -> [_ _]
          tunnel: w231 -> [w239 w257]
          tunnel: [w238 w256] -> w230
          tunnel: ["Avg Current" ("Lable.Unit_VOl_MA_UA") "Avg Voltage" ("Lable.Unit_VOl_MA_UA")] -> w229
          tunnel: [T3."Enabled" ("Disabled") T3."Disabled and Grayed Out" ("Disabled")] -> w227
          frame False {
            n169 = flat-sequence {
              tunnel: w239 -> [w242]
              frame #0 {
                n170 = local read "Task out"() -> (w240:refnum<k21>)
                n171 = call "uA_daq_Clear_usb_DAQ.vi"("Refnum in"=w240) -> ()  [unwired: 11 in]
              }
              frame #1 {
                n172 = call "uA_daq_ON_OFF_LED_Measure.vi"("LED_meas"=FALSE ("Boolean"), "USB"=w242) -> ()  [unwired: 9 in, 1 out]
              }
              frame #2 {
                n173 = local write "Task out"(refnum<k21> "Stop" ("Refnum out")) -> ()
              }
            }
          }
          frame True {
            w255 = "V" ("Y Scale.Name Label.Text")
            n174 = local read "Sampling Rate"() -> (w247:T1)
            n175 = property on="Waveform_main" class="WFGraph (strict)"("YScale.NameLbl.Text"=w255) -> (error out=w252:errorcluster)  [unwired: 2 in, 1 out]
            n176 = call "Sample rate to sample collected.vi"("Sampling Rate _menu"=w247) -> ("Sample_rate"=w246:u32, "Sample"=w248:i32)  [unwired: 9 in]
            n177 = local write "Samples"(w248) -> ()
            n178 = property on="Waveform_sub" class="WFGraph (strict)"(error in=w252, "YScale.NameLbl.Text"=w255) -> (error out=w253:errorcluster)  [unwired: 1 in, 1 out]
            n179 = local read "Task out"() -> (w258:refnum<k21>)
            n180 = property on="Waveform_main" class="WFGraph (strict)"(error in=w253, "YScale.Maximum"=5.0 ("Y Scale.Range:Maximum")) -> ()  [unwired: 1 in, 2 out]
            n181 = call "UEvent_MONITOR_VBAT.vi"("Vout  - Vbat profile"=enum16{"3.8VDC", "2.9VDC", "By Pass", "4.0VDC"}."By Pass", "Sample rate"=w246, "USB"=w257, "Range - Shunts"=Range_Shunt_selector."mA Range Rs = 1ohm", "Refnum in"=w258) -> ("Refnum out"=w250:refnum<k21>, "Power ON/OFF"=w259:bool)  [unwired: 1 in, 4 out]
            n182 = local write "Power ON/OFF"(w259) -> ()
            n183 = local write "Task out"(w250) -> ()
          }
        }
        n184 = Request Deallocation(TRUE ("flag")) -> ()
        n185 = property on="Range - Shunts" class="Enum (strict)"("DisabledEnum"=w227) -> ()  [unwired: 2 in, 2 out]
        n186 = property on="Lable.Unit_VOl_MA_UA" class="Str"("Value"=w229) -> ()  [unwired: 2 in, 2 out]
        n187 = property on="Measure" class="Bool (strict)"("Value"=w230) -> ()  [unwired: 2 in, 2 out]
      }
      event "Vout  - Vbat profile": Value Change {
        n188 = event-data() -> ()  [unwired: 1 in, 6 out]
        n189 = Not Equal?(x="Vout  - Vbat profile", y=enum16{"3.8VDC", "2.9VDC", "By Pass", "4.0VDC"}."2.9VDC" ("Vout  - Vbat profile")) -> (x != y?=w272:bool)
        n190 = case shown="True" w272 {
          tunnel: [w283 w284] -> w270
          tunnel: FALSE -> [w283 _]
          frame False {
          }
          frame True {
            n191 = property on="Profile" class="Enum (strict)"() -> ("Value"=w286:enum16{"SAM", "DIANA", "Hi-POWER", "Other..."})  [unwired: 2 in, 2 out]
            n192 = Equal?(x=w286, y=enum16{"SAM", "DIANA", "Hi-POWER", "Other..."}."SAM" ("Profile")) -> (x = y?=w284:bool)
          }
        }
        n193 = call "Display Message to User"("Enable"=w270) -> ("OK"=w269:bool)  [unwired: 9 in, 1 out]
        n194 = case shown="False" w269 {
          tunnel: [w281 w282] -> w266
          tunnel: "Vout  - Vbat profile" -> [w281 _]
          frame False {
          }
          frame True {
            w282 = enum16{"3.8VDC", "2.9VDC", "By Pass", "4.0VDC"}."2.9VDC" ("Vout  - Vbat profile")
            n195 = property on="Vout  - Vbat profile" class="Enum (strict)"("Value"=w282) -> ()  [unwired: 2 in, 2 out]
          }
        }
        n196 = case shown="\"4.0VDC\"" w266 {
          tunnel: [3.8 2.9 99.0 4.0] -> w262
          tunnel: [TRUE ("Visible") TRUE ("Visible") FALSE ("Visible") TRUE ("Visible")] -> _
          frame "3.8VDC", Default {
          }
          frame "2.9VDC" {
          }
          frame "By Pass" {
          }
          frame "4.0VDC" {
          }
        }
        n197 = Number To Fractional String(number=w262, width (-)=i16 1, precision (6)=i16 1) -> (F-format string=w265:string)  [unwired: 1 in]
        n198 = Concatenate Strings("LDO: " ("string"), w265, "V" ("string")) -> ()  [unwired: 1 out]
      }
      event "Internal PW": Value Change {
        n199 = event-data() -> ()  [unwired: 1 in, 6 out]
        n200 = local read "Sampling Rate"() -> (w289:T1)
        n201 = case shown="True" "Internal PW" {
          tunnel: [T5."Internal PW Source" ("Ex/Int PW") T5."External PW Source" ("Ex/Int PW")] -> w301
          frame False {
            # "Internal power source"
          }
          frame True {
            # "External Power Source"
          }
        }
        n202 = property on="Ext PW Vol Monitor" class="Bool (strict)"() -> ("Value"=w297:bool)  [unwired: 2 in, 2 out]
        n203 = property on="Range - Shunts" class="Enum (strict)"() -> ("Value"=w300:T2)  [unwired: 2 in, 2 out]
        n204 = local read "Task out"() -> (w304:refnum<k21>)
        n205 = local read "USB"() -> (w299:tag)
        n206 = call "Sample rate to sample collected.vi"("Sampling Rate _menu"=w289) -> ("Sample_rate"=w287:u32, "Sample"=w288:i32)  [unwired: 9 in]
        n207 = local write "Samples"(w288) -> ()
        n208 = call "UEvent_SET_INTERNAL_EXTERNAL_POWER_SOURCE.vi"("Ex/Int PW"=w301, "Sample rate"=w287, "Ext PW Vol Monitor"=w297, "USB"=w299, "Value"=w300, "Refnum in"=w304) -> ("External Voltage HIGH"=w296:bool, "Battery_Voltage"=w303:dbl, "DUT_Voltage"=w302:dbl, "Refnum out"=w298:refnum<k21>)  [unwired: 2 in]
        n209 = local read "Measure"() -> (w295:bool)
        n210 = case shown="True" w296 {
          tunnel: w296 -> [_ w312]
          tunnel: [w311 w312] -> w291
          tunnel: "Internal PW" -> [w311 _]
          frame True {
          }
          frame False {
            n211 = property on="Internal PW" class="Bool (strict)"("Value"=w312) -> ()  [unwired: 2 in, 2 out]
          }
        }
        n212 = local write "PW_Internal_Source"(w303) -> ()
        n213 = local write "Vbat"(w302) -> ()
        n214 = case shown="False" w295 {
          tunnel: w298 -> [_ w310]
          tunnel: [refnum<k21> "Stop" ("Refnum out") w310] -> w294
          frame False {
          }
          frame True {
          }
        }
        n215 = local read "Vout  - Vbat profile"() -> (w292:enum16{"3.8VDC", "2.9VDC", "By Pass", "4.0VDC"})
        n216 = local write "Task out"(w294) -> ()
        n217 = local write "EX_IN_INdicator"(w291) -> ()
        n218 = Not(x=w291) -> (.not. x?=w290:bool)
        n219 = case shown="\"By Pass\"" w292 {
          tunnel: w290 -> [w305 w306 _ w308]
          tunnel: [w305 w306 FALSE w308] -> _
          frame "3.8VDC", Default {
          }
          frame "2.9VDC" {
          }
          frame "By Pass" {
          }
          frame "4.0VDC" {
          }
        }
        "PW_Source" <- "Internal PW"
      }
      event "bypass Shunt": Value Change {
        n220 = event-data() -> ()  [unwired: 1 in, 6 out]
        n221 = Not(x="bypass Shunt") -> (.not. x?=w324:bool)
        n222 = local read "Sampling Rate"() -> (w316:T1)
        n223 = case shown="True" "bypass Shunt" {
          tunnel: [T6."Turn Off bypass - On Shunt" ("Bypass Shunt") T6."Turn On bypass - Off Shunt" ("Bypass Shunt")] -> w328
          frame False {
            # "add Shunt"
          }
          frame True {
            # "No Shunt"
          }
        }
        n224 = property on="schematic" class="Bool (strict)"("Value"=w324) -> ()  [unwired: 2 in, 2 out]
        n225 = property on="Ext PW Vol Monitor" class="Bool (strict)"() -> ("Value"=w322:bool)  [unwired: 2 in, 2 out]
        n226 = local read "Task out"() -> (w325:refnum<k21>)
        n227 = local read "USB"() -> (w327:tag)
        n228 = call "Sample rate to sample collected.vi"("Sampling Rate _menu"=w316) -> ("Sample_rate"=w315:u32, "Sample"=w317:i32)  [unwired: 9 in]
        n229 = local write "Samples"(w317) -> ()
        n230 = property on="Range - Shunts" class="Enum (strict)"() -> ("Value"=w326:T2)  [unwired: 2 in, 2 out]
        n231 = call "UEvent_SET_BYPASS_SHUNT_OR_NOT.vi"("Sample rate"=w315, "Task in"=w325, "Ext PW Vol Monitor"=w322, "USB"=w327, "Bypass Shunt"=w328, "Range_shunt"=w326) -> ("error out"=→"error out 3":errorcluster, "Task out"=w319:refnum<k21>)  [unwired: 4 in]
        n232 = local read "Measure"() -> (w321:bool)
        n233 = local write "Task out"(w319) -> ()
        n234 = case shown="False" w321 {
          tunnel: w319 -> [_ w330]
          tunnel: [refnum<k21> "Stop" ("Refnum out") w330] -> w320
          frame False {
          }
          frame True {
          }
        }
        n235 = local write "Task out"(w320) -> ()
      }
      event "Power ON/OFF": Value Change {
        n236 = event-data() -> ()  [unwired: 1 in, 6 out]
        n237 = case shown="False" "Power ON/OFF" {
          tunnel: [enum16{"Power ON DUT", "Power OFF DUT"}."Power OFF DUT" ("Power ON/OFF DUT") enum16{"Power ON DUT", "Power OFF DUT"}."Power ON DUT" ("Power ON/OFF DUT")] -> w345
          frame False {
          }
          frame True {
            # "ON"
          }
        }
        n238 = local read "Sampling Rate"() -> (w334:T1)
        n239 = local read "Vout  - Vbat profile"() -> (w344:enum16{"3.8VDC", "2.9VDC", "By Pass", "4.0VDC"})
        n240 = property on="Ext PW Vol Monitor" class="Bool (strict)"() -> ("Value"=w340:bool)  [unwired: 2 in, 2 out]
        n241 = property on="Range - Shunts" class="Enum (strict)"() -> ("Value"=w343:T2)  [unwired: 2 in, 2 out]
        n242 = local read "Task out"() -> (w347:refnum<k21>)
        n243 = local read "USB"() -> (w342:tag)
        n244 = call "Sample rate to sample collected.vi"("Sampling Rate _menu"=w334) -> ("Sample_rate"=w333:u32, "Sample"=w335:i32)  [unwired: 9 in]
        n245 = local write "Samples"(w335) -> ()
        n246 = call "UEvent_ON_OFF_POWER_SOURCE.vi"("Sample rate"=w333, "USB"=w342, "Power ON/OFF DUT"=w345, "Ext PW Vol Monitor"=w340, "Value"=w343, "Vout  - Vbat profile"=w344, "Refnum in"=w347) -> ("Battery_Voltage"=w346:dbl, "DUT_Voltage"=w336:dbl, "Refnum out"=w337:refnum<k21>)  [unwired: 2 in]
        n247 = local read "Measure"() -> (w339:bool)
        n248 = local write "PW_Internal_Source"(w346) -> ()
        n249 = local write "Vbat"(w336) -> ()
        n250 = local write "vbat_lb"(w336) -> ()
        n251 = local write "Task out"(w337) -> ()
        n252 = case shown="False" w339 {
          tunnel: w337 -> [_ w349]
          tunnel: [refnum<k21> "Stop" ("Refnum out") w349] -> w338
          frame False {
          }
          frame True {
          }
        }
        n253 = local write "Task out"(w338) -> ()
        "POWER ON_OFF" <- "Power ON/OFF"
      }
      event "Profile": Value Change {
        n254 = event-data() -> ()  [unwired: 1 in, 6 out]
        n255 = case shown="\"Hi-POWER\"" "Profile" {
          tunnel: [enum16{"3.8VDC", "2.9VDC", "By Pass", "4.0VDC"}."2.9VDC" ("DUT Voltage Selector") enum16{"3.8VDC", "2.9VDC", "By Pass", "4.0VDC"}."By Pass" ("DUT Voltage Selector") enum16{"3.8VDC", "2.9VDC", "By Pass", "4.0VDC"}."3.8VDC" ("DUT Voltage Selector") enum16{"3.8VDC", "2.9VDC", "By Pass", "4.0VDC"}."By Pass" ("DUT Voltage Selector")] -> w352
          frame "SAM", Default {
          }
          frame "Other..." {
          }
          frame "DIANA" {
          }
          frame "Hi-POWER" {
          }
        }
        n256 = local write "Vout  - Vbat profile"(w352) -> ()
      }
      event "Waveform_main": Cursor Move {
        n257 = event-data() -> ()  [unwired: 1 in, 9 out]
        n258 = local read "Waveform_main"() -> (w366:waveform(sgl))
        n259 = property on="Waveform_main" class="WFGraph (strict)"() -> ("CrsrList"=w376:T7)  [unwired: 2 in, 2 out]
        n260 = local read "Sampling Rate"() -> (w359:T1)
        n261 = call "Sample rate to sample collected.vi"("Sampling Rate _menu"=w359) -> ("Sample_rate"=w358:u32)  [unwired: 9 in, 1 out]
        n262 = call "uA_daq_Capture_Current_waveform_to_new_chart.vi"("Sample rate"=w358, "CrsrList"=w376, "Waveform_main"=w366) -> ("Numeric"=w373:dbl, "Waveform"=w374:waveform(sgl), "Numeric 2"=w375:sgl)  [unwired: 6 in]
        n263 = local write "Avg"(w375) -> ()
        n264 = local write "Waveform_sub"(w374) -> ()
        n265 = property on="Waveform_sub" class="WFGraph (strict)"("XScale.Maximum"=w373, "XScale.Minimum"=0.0 ("X Scale.Range:Minimum")) -> (error out=w360:errorcluster)  [unwired: 2 in, 1 out]
        n266 = property on="Waveform_main" class="WFGraph (strict)"(error in=w360, "Active Cursor"=u32 1) -> (error out=w368:errorcluster, "Value"=w367:waveform(sgl), "Cursor.Cursor X"=w370:dbl)  [unwired: 1 in, 1 out]
        n267 = property on="Waveform_main" class="WFGraph (strict)" props=["CrsrList", "Active Cursor", "Cursor", "Cursor X"](error in=w368, "Active Cursor"=u32 0) -> ("Cursor.Cursor X"=w369:dbl)  [unwired: 1 in, 3 out]
        n268 = call "uA_daq_calculate_All_values_from Sub_chart.vi"("Cursor.Cursor X 2"=w370, "Cursor.Cursor X"=w369, "Value"=w367, "Sample rate"=w358) -> ("Max value"=→"Max":dbl, "Average"=→"Avg":dbl, "Delta(s)"=→"Delta(s)":sgl, "Min value"=→"Min":dbl)  [unwired: 3 in, 1 out]
      }
      event "Calib": Value Change {
        w382 = Range_Shunt_selector."uA Range  Rs = 3.3ohm" ("Range - Shunts")
        n269 = event-data() -> ()  [unwired: 1 in, 6 out]
        n270 = call "Display Message to User2"() -> ("error out"=w378:errorcluster)  [unwired: 10 in, 1 out]
        n271 = flat-sequence {
          tunnel: w378 -> [_]
          tunnel: [w442] -> w380
          tunnel: [w437] -> w381
          frame #0 {
            n272 = local write "Measure"(FALSE ("Measure")) -> ()
          }
          frame #1 {
            n273 = local read "Task out"() -> (w437:refnum<k21>)
            n274 = local write "Waveform_main"(waveform(sgl) {"t0"=timestamp(0 s since 1904-01-01), "dt"=1.0, "Y"=[]} ("Waveform_main")) -> ()
            n275 = Wait (ms)(milliseconds to wait=u32 1000) -> ()  [unwired: 1 out]
            n276 = local write "uA_bank0"(0.0 ("uA_bank0")) -> ()
            n277 = call <vilib>:"DAQmx Stop Task.vi"("task/channels in"=w437) -> ("task out"=w439:refnum<k21>, "error out"=w440:errorcluster)  [unwired: 13 in]
            n278 = call <vilib>:"DAQmx Clear Task.vi"("task in"=w439, "error in"=w440) -> ("error out"=w438:errorcluster)  [unwired: 13 in]
            n279 = local read "USB"() -> (w442:tag)
            n280 = case shown="Error" w438 {
              frame No Error {
                n281 = local write "Task out"(refnum<k21> "Stop" ("y")) -> ()
              }
              frame Error {
              }
            }
          }
        }
        n282 = call "UEvent_MEASURE_FULL_PROCESS_START.vi"("Refnum in"=w381, "Range - Shunts"=w382, "Ext PW Vol Monitor"=FALSE, "USB"=w380, "Internal/external Power"=FALSE) -> ("Refnum out"=w384:refnum<k21>, "error out"=w385:errorcluster)  [unwired: 4 in, 5 out]
        n283 = while {
          tunnel: w385 -> [w429]
          tunnel: w384 -> [w431]
          tunnel: [w429] -> w383
          stop <- TRUE stop-if-true
          n284 = local write "Task out"(w431) -> ()
          n285 = local write "Measure"(TRUE ("Measure")) -> ()
          n286 = Wait (ms)(milliseconds to wait=u32 10000) -> ()  [unwired: 1 out]
        }
        n287 = flat-sequence {
          tunnel: w383 -> [w424]
          tunnel: w382 -> [w425]
          tunnel: [w424] -> w379
          frame #0 {
            n288 = local read "Average (uA)"() -> (w427:dbl)
            n289 = local read "DEV SN"() -> (w426:u32)
            n290 = local write "Measure"(FALSE ("Measure")) -> ()
            n291 = local write "uA_bank0"(w427) -> ()
            n292 = call "Calibration_Save_file.vi"("Current"=w427, "Range - Shunts"=w425, "DEV SN"=w426) -> ()  [unwired: 8 in, 1 out]
          }
        }
        n293 = flat-sequence {
          tunnel: w379 -> [w394]
          tunnel: [w394] -> w390
          tunnel: [w393] -> w389
          tunnel: [w392] -> w388
          tunnel: [Range_Shunt_selector."mA Range Rs = 1ohm" ("Range - Shunts")] -> w377
          tunnel: w390 -> [_]
          tunnel: w389 -> [w409]
          tunnel: w388 -> [w408]
          tunnel: w377 -> [w406]
          frame #0 {
            n294 = flat-sequence {
              tunnel: [w404] -> w392
              tunnel: [w399] -> w393
              frame #0 {
                n295 = local write "Measure"(FALSE ("Measure")) -> ()
                n296 = Wait (ms)(milliseconds to wait=u32 1000) -> ()  [unwired: 1 out]
              }
              frame #1 {
                n297 = local read "Task out"() -> (w399:refnum<k21>)
                n298 = local read "USB"() -> (w404:tag)
                n299 = local write "Waveform_main"(waveform(sgl) {"t0"=timestamp(0 s since 1904-01-01), "dt"=1.0, "Y"=[]} ("Waveform_main")) -> ()
                n300 = Wait (ms)(milliseconds to wait=u32 2000) -> ()  [unwired: 1 out]
                n301 = local write "mARange"(0.0 ("uA_bank0")) -> ()
                n302 = call <vilib>:"DAQmx Stop Task.vi"("task/channels in"=w399) -> ("task out"=w401:refnum<k21>, "error out"=w402:errorcluster)  [unwired: 13 in]
                n303 = call <vilib>:"DAQmx Clear Task.vi"("task in"=w401, "error in"=w402) -> ("error out"=w400:errorcluster)  [unwired: 13 in]
                n304 = case shown="No Error" w400 {
                  frame No Error {
                    n305 = local write "Task out"(refnum<k21> "Stop" ("y")) -> ()
                  }
                  frame Error {
                  }
                }
              }
            }
          }
          frame #1 {
            n306 = property on="Range - Shunts" class="Enum (strict)"("Value"=w406) -> ()  [unwired: 2 in, 2 out]
            n307 = call "UEvent_MEASURE_FULL_PROCESS_START.vi"("Refnum in"=w409, "Range - Shunts"=w406, "Ext PW Vol Monitor"=FALSE, "USB"=w408, "Internal/external Power"=TRUE) -> ("Refnum out"=w411:refnum<k21>, "error out"=w410:errorcluster)  [unwired: 4 in, 5 out]
            n308 = while {
              tunnel: w410 -> [w419]
              tunnel: w411 -> [w421]
              tunnel: [w419] -> w407
              stop <- TRUE stop-if-true
              n309 = local write "Task out"(w421) -> ()
              n310 = local write "Measure"(TRUE ("Measure")) -> ()
              n311 = Wait (ms)(milliseconds to wait=u32 5000) -> ()  [unwired: 1 out]
            }
            n312 = flat-sequence {
              tunnel: w407 -> [w414]
              tunnel: w406 -> [w415]
              frame #0 {
                n313 = local read "Average (uA)"() -> (w416:dbl)
                n314 = local write "Measure"(FALSE ("Measure")) -> ()
                n315 = local read "DEV SN"() -> (w417:u32)
                n316 = local write "mARange"(w416) -> ()
                n317 = call "Calibration_Save_file.vi"("Current"=w416, "error in (no error)"=w414, "Range - Shunts"=w415, "DEV SN"=w417) -> ()  [unwired: 7 in, 1 out]
              }
            }
          }
          frame #2 {
            n318 = call "Display Message to User3"() -> ()  [unwired: 10 in, 2 out]
          }
        }
      }
      event "Clear Graph": Value Change {
        n319 = event-data() -> ()  [unwired: 1 in, 6 out]
        n320 = flat-sequence {
          frame #0 {
            w444 = waveform(sgl) {"t0"=timestamp(0 s since 1904-01-01), "dt"=1.0, "Y"=[]} ("Waveform_main")
            n321 = local write "Clear"(TRUE ("Clear")) -> ()
            n322 = Wait (ms)(milliseconds to wait=u32 500) -> ()  [unwired: 1 out]
            n323 = local write "Waveform_main"(w444) -> ()
            n324 = local write "Waveform_sub"(w444) -> ()
          }
          frame #1 {
            n325 = local write "Clear"(FALSE ("Clear")) -> ()
          }
        }
      }
      event "ZOOM +": Value Change {
        n326 = event-data() -> ()  [unwired: 1 in, 6 out]
        n327 = property on="Waveform_main" class="WFGraph (strict)" props=["XScale", "Range", "XScale", "Increment", "XScale", "Maximum", "XScale", "Minimum"]() -> ("XScale.Maximum"=w453:dbl, "XScale.Minimum"=w449:dbl)  [unwired: 2 in, 4 out]
        n328 = Subtract(x=w453, y=0.1) -> (x-y=w451:dbl)
        n329 = Add(x=w449, y=0.1) -> (x+y=w448:dbl)
        n330 = property on="Waveform_main" class="WFGraph (strict)"("XScale.Maximum"=w451, "XScale.Minimum"=w448) -> ()  [unwired: 2 in, 2 out]
      }
      event "ZOOM -": Value Change {
        n331 = event-data() -> ()  [unwired: 1 in, 6 out]
        n332 = property on="Waveform_main" class="WFGraph (strict)" props=["XScale", "Range", "XScale", "Increment", "XScale", "Maximum", "XScale", "Minimum"]() -> ("XScale.Maximum"=w462:dbl, "XScale.Minimum"=w458:dbl)  [unwired: 2 in, 4 out]
        n333 = Add(x=w462, y=0.1) -> (x+y=w460:dbl)
        n334 = Subtract(x=w458, y=0.1) -> (x-y=w455:dbl)
        n335 = Less Than 0?(x=w455) -> (x < 0?=w457:bool)
        n336 = Select(t=0.0, s=w457, f=w455) -> (s? t:f=w454:dbl)
        n337 = property on="Waveform_main" class="WFGraph (strict)"("XScale.Maximum"=w460, "XScale.Minimum"=w454) -> ()  [unwired: 2 in, 2 out]
      }
      event "ZOOM M1M2": Value Change {
        n338 = event-data() -> ()  [unwired: 1 in, 6 out]
        n339 = property on="Waveform_main" class="WFGraph (strict)"("Active Cursor"=u32 0) -> (error out=w469:errorcluster)  [unwired: 2 in, 1 out]
        n340 = property on="Waveform_main" class="WFGraph (strict)"(error in=w469) -> (error out=w466:errorcluster, "Cursor.Cursor X"=w464:dbl)  [unwired: 1 in, 1 out]
        n341 = property on="Waveform_main" class="WFGraph (strict)"(error in=w466, "Active Cursor"=u32 1) -> (error out=w468:errorcluster)  [unwired: 1 in, 1 out]
        n342 = property on="Waveform_main" class="WFGraph (strict)"(error in=w468) -> ("Cursor.Cursor X"=w463:dbl)  [unwired: 1 in, 2 out]
        n343 = Greater?(x=w464, y=w463) -> (0:w465:bool)
        n344 = case shown="True" w465 {
          tunnel: w464 -> [w472 w474]
          tunnel: w463 -> [w471 w473]
          frame False {
            n345 = property on="Waveform_main" class="WFGraph (strict)"("XScale.Maximum"=w471, "XScale.Minimum"=w472) -> ()  [unwired: 2 in, 2 out]
          }
          frame True {
            n346 = property on="Waveform_main" class="WFGraph (strict)"("XScale.Maximum"=w474, "XScale.Minimum"=w473) -> ()  [unwired: 2 in, 2 out]
          }
        }
      }
      event "Center": Value Change {
        n347 = event-data() -> ()  [unwired: 1 in, 6 out]
        n348 = property on="Waveform_main" class="WFGraph (strict)"() -> ("XScale.Maximum"=w479:dbl, "XScale.Minimum"=w478:dbl)  [unwired: 2 in, 2 out]
        n349 = Add(x=w479, y=w478) -> (x+y=w477:dbl)
        n350 = Divide(x=w477, y=2.0) -> (x/y=w475:dbl)
        n351 = property on="Waveform_main" class="WFGraph (strict)" props=["Value", "Active Cursor", "Cursor", "Cursor X"]("Active Cursor"=u32 1, "Cursor.Cursor X"=w475) -> (error out=w480:errorcluster)  [unwired: 2 in, 2 out]
        n352 = property on="Waveform_main" class="WFGraph (strict)" props=["CrsrList", "Active Cursor", "Cursor", "Cursor X"](error in=w480, "Active Cursor"=u32 0, "Cursor.Cursor X"=w475) -> ()  [unwired: 1 in, 3 out]
      }
      event "stop": Value Change {
        n353 = event-data() -> ()  [unwired: 1 in, 6 out]
        n354 = flat-sequence {
          tunnel: [w487] -> w483
          tunnel: w483 -> [w496]
          frame #0 {
            n355 = local write "Task out"(refnum<k21> "Stop" ("Task out")) -> ()
          }
          frame #1 {
            n356 = local read "USB"() -> (w495:tag)
            n357 = local read "Task out"() -> (w490:refnum<k21>)
            n358 = call "uA_daq_Set_Relay_internal_power_on_off_from_baterry.vi"("Power ON/OFF DUT"=enum16{"Power ON DUT", "Power OFF DUT"}."Power OFF DUT", "USB DAQ"=w495) -> ("error out"=w486:errorcluster)  [unwired: 9 in]
            n359 = call <vilib>:"DAQmx Stop Task.vi"("task/channels in"=w490, "error in"=w486) -> ("task out"=w485:refnum<k21>, "error out"=w488:errorcluster)  [unwired: 12 in]
            n360 = call <vilib>:"DAQmx Clear Task.vi"("task in"=w485, "error in"=w488) -> ("error out"=w489:errorcluster)  [unwired: 13 in]
            n361 = local read "USB"() -> (w493:tag)
            n362 = call <vilib>:"Clear Errors.vi"("error in (no error)"=w489) -> ("error out"=w492:errorcluster)  [unwired: 5 in, 1 out]
            n363 = call "uA_daq_ON_OFF_LED_Measure.vi"("error in"=w492, "LED_meas"=FALSE ("Boolean"), "USB"=w493) -> ("error out"=w487:errorcluster)  [unwired: 8 in]
          }
          frame #2 {
            n364 = local read "Ver"() -> (w497:string)
            n365 = call <vilib>:"Clear Errors.vi"("error in (no error)"=w496) -> ()  [unwired: 5 in, 2 out]
            n366 = Empty String/Path?(string/path=w497) -> (empty?=w498:bool)
            n367 = case shown="False" w498 {
              frame True {
              }
              frame False {
                n368 = Quit LabVIEW(quit? (T)=TRUE) -> ()
              }
            }
          }
          frame #3 {
            n369 = Stop(stop? (T)=TRUE) -> ()
          }
        }
      }
      event "Save": Value Change {
        n370 = event-data() -> ()  [unwired: 1 in, 6 out]
        n371 = local read "Waveform_main"() -> (w502:waveform(sgl))
        n372 = call "File Dialog"("pattern (all files)"="*.dlog", "pattern label"="datalog") -> ("selected path"=w505:path)  [unwired: 10 in, 3 out]
        n373 = call-poly <vilib>:"Write Waveforms to File.vi"("append to file? (new file:F)"=FALSE, "waveform"=w502, "file path (dialog if empty)"=w505) -> ()  [unwired: 7 in, 2 out]
      }
      event "Load": Value Change {
        (unwired) FALSE ("append to file? (new file:F)")
        n374 = event-data() -> ()  [unwired: 1 in, 6 out]
        n375 = call "File Dialog3"("pattern (all files)"="*.dlog", "pattern label"="datalog") -> ("selected path"=w509:path)  [unwired: 10 in, 3 out]
        n376 = call-poly <vilib>:"Read Waveforms from File.vi"("file path (dialog if empty)"=w509) -> ("first waveform in record"=w506:waveform(dbl))  [unwired: 5 in, 3 out]
        n377 = local write "Waveform_main"(w506) -> ()
      }
      event "Take Picture": Value Change {
        n378 = event-data() -> ()  [unwired: 1 in, 6 out]
        n379 = call <vilib>:"Application Directory.vi"() -> ("Application Directory"=w511:path)
        n380 = control-ref of="This VI"() -> (w515:refnum<vi>)
        n381 = call "File Dialog2"("start path"=w511, "pattern (all files)"="*.jpg", "pattern label"="*.jpg") -> ("selected path"=w517:path, "error out"=w514:errorcluster)  [unwired: 9 in, 2 out]
        n382 = invoke on="Invoke Node" class="VI" method="FP.Get Image"(reference=w515, "image depth"=enum32{"File", "Clipboard"}."File" ("Target")) -> ("image data"=w516:T8)  [unwired: 4 in, 5 out]
        n383 = call <vilib>:"Clear Errors.vi"("error in (no error)"=w514) -> ()  [unwired: 5 in, 2 out]
        n384 = call <vilib>:"Write JPEG File.vi"("image data"=w516, "path to JPEG file"=w517) -> ()  [unwired: 8 in, 2 out]
      }
      event "Save setting": Value Change {
        w539 = "SETTING" ("section")
        n385 = event-data() -> ()  [unwired: 1 in, 6 out]
        n386 = call <vilib>:"Application Directory.vi"() -> ("Application Directory"=w544:path)
        n387 = local read "Range - Shunts"() -> (w532:T2)
        n388 = Build Path(base path=w544, name or relative path="Setting.cfg") -> (appended path=w542:path)
        n389 = local read "Vout  - Vbat profile"() -> (w529:enum16{"3.8VDC", "2.9VDC", "By Pass", "4.0VDC"})
        n390 = call <vilib>:"Open Config Data.vi"("create file if necessary (T)"=TRUE, "configuration file path"=w542) -> ("error out"=w518:errorcluster, "refnum"=w540:T4)  [unwired: 7 in, 1 out]
        n391 = local read "Profile"() -> (w531:enum16{"SAM", "DIANA", "Hi-POWER", "Other..."})
        n392 = call-poly <vilib>:"Write Key.vi"("section"=w539, "error in (no error)"=w518, "value"=w532, "key"="Range - Shunts", "refnum"=w540) -> ("error out"=w519:errorcluster, "refnum out"=w537:T4)  [unwired: 4 in, 1 out]
        n393 = local read "Internal PW"() -> (w527:bool)
        n394 = call-poly <vilib>:"Write Key.vi"("section"=w539, "error in (no error)"=w519, "value"=w531, "key"="Profile", "refnum"=w537) -> ("error out"=w520:errorcluster, "refnum out"=w538:T4)  [unwired: 4 in, 1 out]
        n395 = local read "bypass Shunt"() -> (w525:bool)
        n396 = call-poly <vilib>:"Write Key.vi"("section"=w539, "error in (no error)"=w520, "value"=w529, "key"="Vout  - Vbat profile", "refnum"=w538) -> ("error out"=w521:errorcluster, "refnum out"=w536:T4)  [unwired: 4 in, 1 out]
        n397 = call-poly <vilib>:"Write Key.vi"("section"=w539, "error in (no error)"=w521, "value"=w527, "key"="Internal PW", "refnum"=w536) -> ("error out"=w522:errorcluster, "refnum out"=w535:T4)  [unwired: 4 in, 1 out]
        n398 = call-poly <vilib>:"Write Key.vi"("section"=w539, "error in (no error)"=w522, "value"=w525, "key"="bypass Shunt", "refnum"=w535) -> ("error out"=w523:errorcluster, "refnum out"=w524:T4)  [unwired: 4 in, 1 out]
        n399 = call <vilib>:"Close Config Data.vi"("error in (no error)"=w523, "refnum"=w524) -> ()  [unwired: 8 in, 2 out]
      }
    }
  }
  n400 = while {
    tunnel: w4 -> [w554]
    tunnel: [w553] -> w7
    shift-right: [w549] -> w6
    shift-left: w5 -> [w551]
    stop <- FALSE ("stop (F)") stop-if-true
    n401 = local read "Range - Shunts"() -> (w548:T2)
    n402 = local read "Samples"() -> (w545:i32)
    n403 = Equal?(x=w551, y=refnum<k21> "Stop") -> (x = y?=w547:bool)
    n404 = case shown="True" w547 {
      tunnel: w554 -> [w557 w565]
      tunnel: [w557 w564] -> w553
      tunnel: w551 -> [_ w561]
      tunnel: [w556 w563] -> w549
      tunnel: w548 -> [_ w562]
      tunnel: refnum<k21> refnum ("task out") -> [_ w559]
      tunnel: w545 -> [_ w558]
      frame True {
        n405 = Wait (ms)(milliseconds to wait=u32 100) -> ()  [unwired: 1 out]
        n406 = local read "Task out"() -> (w556:refnum<k21>)
      }
      frame False {
        n407 = Not Equal?(x=w561, y=w559) -> (x != y?=w560:bool)
        n408 = case shown="True" w560 {
          tunnel: w565 -> [w567 w573]
          tunnel: [w567 w572] -> w564
          tunnel: w561 -> [_ w571]
          tunnel: [w566 w570] -> w563
          tunnel: w562 -> [_ w569]
          tunnel: w558 -> [_ w568]
          frame False {
            n409 = local read "Task out"() -> (w566:refnum<k21>)
          }
          frame True {
            n410 = case shown="\"mA Range Rs = 1ohm\"" w569 {
              tunnel: w573 -> [w580 w591 w602 w613]
              tunnel: [w579 w590 w601 w612] -> w572
              tunnel: w571 -> [w578 w589 w600 w611]
              tunnel: [w577 w588 w599 w610] -> w570
              tunnel: w568 -> [w574 w585 w596 w607]
              frame "mA Range Rs = 1ohm" {
                n411 = call "DAQ_ADC_Max_Sample_Rate_For_USB_6001.vi"("number of samples per channel"=w574, "Refnum in"=w578) -> ("error out"=w576:errorcluster, "data"=w575:waveform(dbl))  [unwired: 8 in]
                n412 = case shown="No Error" w576 {
                  selector: w576 -> [_ w584]
                  tunnel: w580 -> [w583 _]
                  tunnel: [w582 _] -> w579
                  tunnel: w575 -> [w581 _]
                  frame No Error {
                    n413 = Enqueue Element(queue=w583, element=w581) -> (queue out=w582:refnum<queue>)  [unwired: 2 in, 2 out]
                  }
                  frame Error {
                    n414 = call <vilib>:"Clear Errors.vi"("error in (no error)"=w584) -> ()  [unwired: 5 in, 2 out]
                  }
                }
                n415 = local read "Task out"() -> (w577:refnum<k21>)
              }
              frame "mA Range Rs = 1ohm - X2" {
                n416 = call "DAQ_ADC_Max_Sample_Rate_For_USB_6001.vi"("number of samples per channel"=w585, "Refnum in"=w589) -> ("error out"=w587:errorcluster, "data"=w586:waveform(dbl))  [unwired: 8 in]
                n417 = case shown="No Error" w587 {
                  selector: w587 -> [_ w595]
                  tunnel: w591 -> [w594 _]
                  tunnel: [w593 _] -> w590
                  tunnel: w586 -> [w592 _]
                  frame No Error {
                    n418 = Enqueue Element(queue=w594, element=w592) -> (queue out=w593:refnum<queue>)  [unwired: 2 in, 2 out]
                  }
                  frame Error {
                    n419 = call <vilib>:"Clear Errors.vi"("error in (no error)"=w595) -> ()  [unwired: 5 in, 2 out]
                  }
                }
                n420 = local read "Task out"() -> (w588:refnum<k21>)
              }
              frame "mA Range Rs = 3.3ohm" {
                n421 = call "DAQ_ADC_Max_Sample_Rate_For_USB_6001.vi"("number of samples per channel"=w596, "Refnum in"=w600) -> ("error out"=w598:errorcluster, "data"=w597:waveform(dbl))  [unwired: 8 in]
                n422 = case shown="No Error" w598 {
                  selector: w598 -> [_ w606]
                  tunnel: w602 -> [w605 _]
                  tunnel: [w604 _] -> w601
                  tunnel: w597 -> [w603 _]
                  frame No Error {
                    n423 = Enqueue Element(queue=w605, element=w603) -> (queue out=w604:refnum<queue>)  [unwired: 2 in, 2 out]
                  }
                  frame Error {
                    n424 = call <vilib>:"Clear Errors.vi"("error in (no error)"=w606) -> ()  [unwired: 5 in, 2 out]
                  }
                }
                n425 = local read "Task out"() -> (w599:refnum<k21>)
              }
              frame "uA Range  Rs = 3.3ohm" {
                n426 = call "DAQ_ADC_Max_Sample_Rate_For_USB_6001.vi"("number of samples per channel"=w607, "Refnum in"=w611) -> ("error out"=w609:errorcluster, "data"=w608:waveform(dbl))  [unwired: 8 in]
                n427 = case shown="No Error" w609 {
                  selector: w609 -> [_ w617]
                  tunnel: w613 -> [w616 _]
                  tunnel: [w615 _] -> w612
                  tunnel: w608 -> [w614 _]
                  frame No Error {
                    n428 = Enqueue Element(queue=w616, element=w614) -> (queue out=w615:refnum<queue>)  [unwired: 2 in, 2 out]
                  }
                  frame Error {
                    n429 = call <vilib>:"Clear Errors.vi"("error in (no error)"=w617) -> ()  [unwired: 5 in, 2 out]
                  }
                }
                n430 = local read "Task out"() -> (w610:refnum<k21>)
              }
            }
          }
        }
      }
    }
  }
  n431 = while {
    tunnel: w4 -> [w625]
    tunnel: w1 -> [w620]
    stop <- FALSE stop-if-true
    n432 = property on="Ext PW Vol Monitor" class="Bool (strict)"() -> ("Value"=w631:bool)  [unwired: 2 in, 2 out]
    n433 = local read "Clear"() -> (w634:bool)
    n434 = property on="Range - Shunts" class="Enum (strict)"() -> ("Value"=w629:T2)  [unwired: 2 in, 2 out]
    n435 = Get Queue Status(queue=w625) -> (queue out=w622:refnum<queue>, error out=w626:errorcluster, # elements in queue=w624:i32)  [unwired: 2 in, 5 out]
    n436 = Dequeue Element(queue=w625, error in (no error)=w626) -> (element=w630:waveform(sgl))  [unwired: 1 in, 3 out]
    n437 = case shown="False" w634 {
      tunnel: [waveform(sgl) {"t0"=timestamp(0 s since 1904-01-01), "dt"=1.0, "Y"=[]} ("Waveform_main") w691] -> w633
      tunnel: w620 -> [_ w689]
      tunnel: [FALSE w688] -> w619
      frame True {
      }
      frame False {
        n438 = local read "Sampling Rate"() -> (w687:T1)
        n439 = local read "Waveform_main"() -> (w691:waveform(sgl))
        n440 = Unbundle By Name(w691) -> ("Y"=w690:sgl[])
        n441 = Array Size(array=w690) -> (size(s)=w686:i32)
        n442 = Greater Or Equal?(x=w686, y=w689) -> (x >= y?=w688:bool)
        n443 = call "Convert  Sample to second.vi"("samples collected"=w686, "Sampling Rate"=w687) -> ("Duration"=→"Total Time":string)  [unwired: 6 in, 3 out]
      }
    }
    n444 = Greater?(x=w624, y=100) -> (0:w621:bool)
    n445 = case shown="\"mA Range Rs = 1ohm\"" w629 {
      tunnel: w630 -> [w640 w644 w648 w652]
      tunnel: [w637 w641 w645 w649] -> w628
      frame "mA Range Rs = 3.3ohm" {
        (unwired) 0.0 ("uA_bank0")
        n446 = call-poly <vilib>:"Basic Averaged DC-RMS.vi"("signal in"=w640) -> ("RMS value"=w638:dbl)  [unwired: 7 in, 3 out]
        n447 = Greater?(x=w638, y=3.5) -> (0:w637:bool)
      }
      frame "uA Range  Rs = 3.3ohm" {
        n448 = call-poly <vilib>:"Basic Averaged DC-RMS.vi"("signal in"=w644) -> ("RMS value"=w642:dbl)  [unwired: 7 in, 3 out]
        n449 = Greater?(x=w642, y=3.5) -> (0:w641:bool)
      }
      frame "mA Range Rs = 1ohm" {
        (unwired) 0.0 ("uA_bank0")
        n450 = call-poly <vilib>:"Basic Averaged DC-RMS.vi"("signal in"=w648) -> ("RMS value"=w646:dbl)  [unwired: 7 in, 3 out]
        n451 = Greater?(x=w646, y=4.0) -> (0:w645:bool)
      }
      frame "mA Range Rs = 1ohm - X2" {
        (unwired) 0.0 ("uA_bank0")
        n452 = call-poly <vilib>:"Basic Averaged DC-RMS.vi"("signal in"=w652) -> ("RMS value"=w650:dbl)  [unwired: 7 in, 3 out]
        n453 = Greater?(x=w650, y=2.0) -> (0:w649:bool)
      }
    }
    n454 = case shown="True" w621 {
      tunnel: w622 -> [_ w636]
      frame False {
      }
      frame True {
        n455 = Flush Queue(queue=w636) -> ()  [unwired: 1 in, 3 out]
      }
    }
    n456 = case shown="True" w631 {
      tunnel: w630 -> [w660 w669]
      tunnel: [w660 w668] -> w618
      tunnel: w628 -> [_ w666]
      tunnel: [FALSE w666] -> w627
      frame True {
        n457 = Unbundle By Name(w660) -> ("Y"=w659:sgl[])
        n458 = Add Array Elements(numeric array=w660) -> (sum=w657:sgl)
        n459 = Array Size(array=w659) -> (size(s)=w658:i32)
        n460 = Divide(x=w657, y=w658) -> (x/y=w654:sgl)
        n461 = Greater?(x=w654, y=6) -> (0:w656:bool)
        n462 = case shown="True" w656 {
          frame False {
          }
          frame True {
            n463 = property on="Internal PW" class="Bool (strict)"("Value"=TRUE ("Internal PW")) -> ()  [unwired: 2 in, 2 out]
            n464 = local read "USB"() -> (w663:tag)
            n465 = call "uA_daq_switch_external_internal_pw_source.vi"("USB DAQ"=w663, "Ex/Int PW"=T5."External PW Source") -> ()  [unwired: 9 in, 1 out]
          }
        }
      }
      frame False {
        n466 = property on="Range - Shunts" class="Enum (strict)"() -> ("Value"=w667:T2)  [unwired: 2 in, 2 out]
        n467 = local read "uA_bank0"() -> (w665:dbl)
        n468 = local read "mARange"() -> (w664:dbl)
        n469 = call "uA_daq_gain_caculator.vi"("Waveform Chart in"=w669, "Calib_value_ uA"=w665, "Calib_mA"=w664, "Range - Shunts"=w667) -> ("Waveform out"=w668:waveform(dbl))  [unwired: 11 in]
      }
    }
    n470 = local read "Measure"() -> (w632:bool)
    n471 = case shown="False" w619 {
      tunnel: w618 -> [_ w674]
      tunnel: w633 -> [_ w673]
      tunnel: w632 -> [w670 w672]
      frame True {
        n472 = case shown="True" w670 {
          frame False {
          }
          frame True {
            n473 = call "Display Message to User4"() -> ()  [unwired: 10 in, 2 out]
          }
        }
        n474 = local write "Measure"(FALSE ("Measure")) -> ()
      }
      frame False {
        n475 = case shown="True" w672 {
          tunnel: w674 -> [_ w678]
          tunnel: w673 -> [_ w680]
          frame False {
          }
          frame True {
            n476 = call "WDT Append Waveforms SGL.vi"("waveform B"=w680, "waveform A"=w678) -> ("waveform out"=→"Waveform_main":waveform(sgl))  [unwired: 8 in, 1 out]
            n477 = local read "Waveform_main"() -> (w681:waveform(sgl))
            n478 = property on="Waveform_main" class="WFGraph (strict)"() -> ("CrsrList"=w682:T7)  [unwired: 2 in, 2 out]
            n479 = local read "Sampling Rate"() -> (w676:T1)
            n480 = call "Sample rate to sample collected.vi"("Sampling Rate _menu"=w676) -> ("Sample_rate"=w675:u32)  [unwired: 9 in, 1 out]
            n481 = call "uA_daq_capture_small_curr_waveform.vi"("Sample rate"=w675, "CrsrList"=w682, "Waveform_main"=w681) -> ("Numeric"=→"Average (uA)":sgl)  [unwired: 8 in]
          }
        }
      }
    }
    n482 = property on="out_range" class="Bool (strict)"("Visible"=w627) -> ()  [unwired: 2 in, 2 out]
  }
  n483 = Release Queue(queue=w7) -> ()  [unwired: 2 in, 3 out]
  n484 = call <vilib>:"DAQmx Clear Task.vi"("task in"=w6) -> ()  [unwired: 14 in, 1 out]
